vi "02 HEWH First-Hour Rating Test SM1.vi"(0 "Equipment":T6={"COM Port"="COM3", "MW100"="MW100", "AG34970"="A-34972A", "Chamber"="WT500"}, 2 "Semiphore":T1, 5 "Degree Setting":dbl=58.0, 7 "Flow rate setting":dbl=3.0, 11 "Error In":errorcluster) -> (15 "Error Out":errorcluster)   [LabVIEW 2012]
uses:
  EquipReferences.ctl
  HEWH Tank Indicator.ctl
  PowerElements.ctl
  <vilib>/Platform/fileVersionInfo.llb/FileVersionInformation.ctl
  GEA2/HEWH_Mode.ctl
  ChannelSettings.ctl
  ValveBankPositions.ctl
  HEWH Error Enumeration.ctl
  Intellifaucet/Intellfaucet Mode.ctl
  Global HEWH.vi
  <vilib>/Utility/file.llb/Write To Spreadsheet File (string).vi
  <vilib>/Analysis/baseanly.llb/Mean (DBL).vi
  <vilib>/Analysis/NI_AALBase.lvlib
panel:
  in  "Tab Control 4":enum32{"Debug Info", "Version Info"}(tab)
  in  "Stop Logging":bool
  in  "Stop":bool
  in  "StopSerial":bool
  out "Serial Data In":string
  out "Computer Name":string
  out "exe?":bool
  out "Local?":bool
  in  "End Time(s)":dbl=3600.0
  in  "TFall":dbl=25.0
  out "Current Draw Start Time":dbl format="%.2f"
  in  "RTD 2 Downspout offset":dbl
  out "COM Port":refnum<visa-resource-name>
  out "Chanel List":string
  out "Label Array":string[](array[string])
  out "FileVersionInfo Out":T2
  out "Calibration Path 2":path
  out "Calibration File Array":dbl[][](array[numeric])
  out "Com Errs":dbl
  out "Voltage":dbl=240.0
  in  "Stop Test":bool
  out "Ver.":string
  out "DrawCount":i32
  out "POWER":T3
  out "t*=0":dbl format="%.2f"
  out "Elapsed Time (sec)":dbl format="%.2f"
  out "STATUS":string
  in  "Help":bool
  out "Current Log Data":string[][](array[string])
  out "Number of Records":i32
  out "Tank Display":T4 {"TC6" format="%.2g"; "TIN" format="%.2g"; "TOUT" format="%.2g"; "Mean" format="%.2f"; "Std Dev" format="%.2f"; "TC5" format="%.2g"; "TC4" format="%.2g"; "TC3" format="%.2g"; "TC2" format="%.2g"; "TC1" format="%.2g"}
  out "First Time":bool=TRUE
  out "Current State":string
  out "MW100":refnum<visa-resource-name>
  in  "Tab Control 2":enum32{"TEST STATUS", "DATA VIEW"}(tab)
  in  "Tab Control":T5(tab)=enum."External Program Controls"
  in  "Read Config File":bool
  in  "Config Filename":string="HEWH First Hour Rating.ini"
  out "Data Array":string[][](array[string])
  in  "Purge Condition TC":enum16{"TC1", "TC2", "TC3", "TC4", "TC5", "TC6"}(ring)
  out "Serial Port Available?":bool
  in  "Cold Water Available?":bool=TRUE
  in  "T3":u32=500
  in  "T2":u32=150
  in  "Work File Directory":path=path "c:/work"
  out "LAN IP Address":string="192.168.25.3"
  out "Init Complete":bool=TRUE
  in  "T1":u32=1000
  in  "T4":u32=60000
  in  "T5":u32=50
  in  "Purge Guard Time(s)":dbl=300.0
  in  "Data Sample Period(10s)":dbl=10.0
  in  "Purge0 Condition TC":enum16{"TC1", "TC2", "TC3", "TC4", "TC5", "TC6"}(ring)
  in  "PurgreTempLimit":dbl=124.0
  in  "Save File Directory":path=path "c:/data"
  out "FileName":path
  out "Use Agilent?":bool
  out "GEA2 HyperData":bool
  in  "Expansion Tank?":bool=TRUE
  out "Mode":T7=enum."HighDemand"
  out "Set Point":u8=140
  in  "Purgre0TempLim":dbl=124.0
  in  "RTD In Band":dbl=5.0
  in  "Calibration Path":path=path "C:/work/CalibrationFile.csv"
  out "Calibration File?":bool
  out "Monitoring Temps Chart":T8(graph)
  out "Tcs 1-6":dbl[](array[numeric])
  in  "Skip Waiting for Temp":bool
  out "SetPoint":dbl
  out "T2(TankSensor)":dbl
  in  "T2_Threshold":dbl=0.5
  out "Purge Guard Time":dbl=120.0
  out "PurgreTempLimit":dbl=127.0
  out "DrawCount":i32
  out "Purgre0TempLim":dbl=127.0
  out "Purge Condition TC":enum16{"TC1", "TC2", "TC3", "TC4", "TC5", "TC6"}(ring)
  out "Downspount Flow":dbl(graph)
  out "Downspout Flow":dbl=3.8899999999999997
  out "Downspout Temp":dbl=76.8
  out "Temp Band(+/- F)":dbl=50.0
  out "Flow rate Adj":dbl=85.11482133995038
  out "Purge Temperature":dbl(graph)
  out "Temp Adj":dbl
  in  "Skip Purge":bool
  in  "Skip Waiting for Cutout":bool
  in  "meant tank lower lim":dbl=130.0
  in  "mean tank upper lim":dbl=140.0
  out "Ave Tank Temp":dbl format="%0.2f"
  out "Tc_1":dbl
  in  "Tc1 UL":dbl=140.0
  in  "Tc1 LL":dbl=130.0
  in  "Skip Waiting for Temp 3":bool
  out "Tcs 1-6, Ave. 3":dbl[](array[numeric])
  out "Temps Chart 2":T9(graph)
  out "T_Ave":dbl
  in  "Temp Decline Hystersis":dbl=0.2
  out "T_Ave_Max":dbl
  out "LastDraw":bool=TRUE
  in  "Begin Draw":bool
  out "RTD OUT":dbl(graph)
  out "Last T*min":dbl
  out "Special Last Draw":bool
  out "Discard Last Draw":bool
  out "T*Ave":dbl
  out "T*min":dbl
  out "M*(Gallons)":dbl
  out "T*max":dbl
  out "FlowMeter During Draw":dbl(graph)
  out "Flow":dbl=3.8899999999999997
  out "RTD_IN Value":dbl
  out "Tin Fault":bool
  out "Temp Adj Draw":dbl
  out "Flow Adj Draw":dbl
  out "Iteration":i32
  out "Drawing":bool=TRUE
  out "ETime":dbl format="%.2f"
  in  "K(0.1)":dbl=0.2
  in  "Flow Adjust Time (3s)":dbl=1.5
  out "WattHours":dbl
  out "Error History":string[](array[string])
  out "Com History":string[](array[string])
  out "Test Data":dbl[][](array[numeric])
  out "Executaion Sequence":string[](array[string])
  out "Error Datalogging":errorcluster={"status"=TRUE, "code"=-1073807346, "source"="VISA Read in Gather Test Data.vi"}
  out "Error Serial":errorcluster
  in  "Tab Control 3":enum32{"Temperature", "Power", "Gallons"}(tab)
  out "Temps":T8(graph) caption="Waveform Chart"
  out "Watt Chart":T10(graph)
  out "Gallons Chart":dbl(graph)
  # "FIRST-HOUR RATING TEST"
  # "Offset added to initial draw for initial value\nin Draw."
  # "wait for purge condition:\npower is off or...\nend of time is near or...\npurge condition tc > purge temp limit \nnote temp limit different between first and subsequent runs."
  # "Wait for Cutout..."
  # "Input relays don't detect that UE or LE are on, and Power reading <\nCompressor LL (0.35 kW currently)"
  # "This draw initiation criterion for heat pump\nwater heaters that use supplemental resistive\nheating, however, shall only apply when\nthe water located above the thermostat at\ncut-out is heated to 135 °F±5 °F (57.2 °C±2.8\n°C)."
  # "WAIT FOR TOP HEATER AND COMP OFF."
  # "T*max is max ave temp"
  # "(For Last Draw, If after 30 sec, T< last tmin, stop and discard measurements, else continue)"
  # "Record output water temp after 15 secs, and at 5 sec intervals thereafter\nMonitor inlet water temp, must be 58 +/- 2 F\nTerminate draw when output temp = T*max -25F, record T*min"
  # "Terminate draw.  Record Tmin*, Tmax*, Tave* and M*"
  # "(For Last Draw, If after 30 sec, T< last tmin, stop and discard measurements, else continue)"
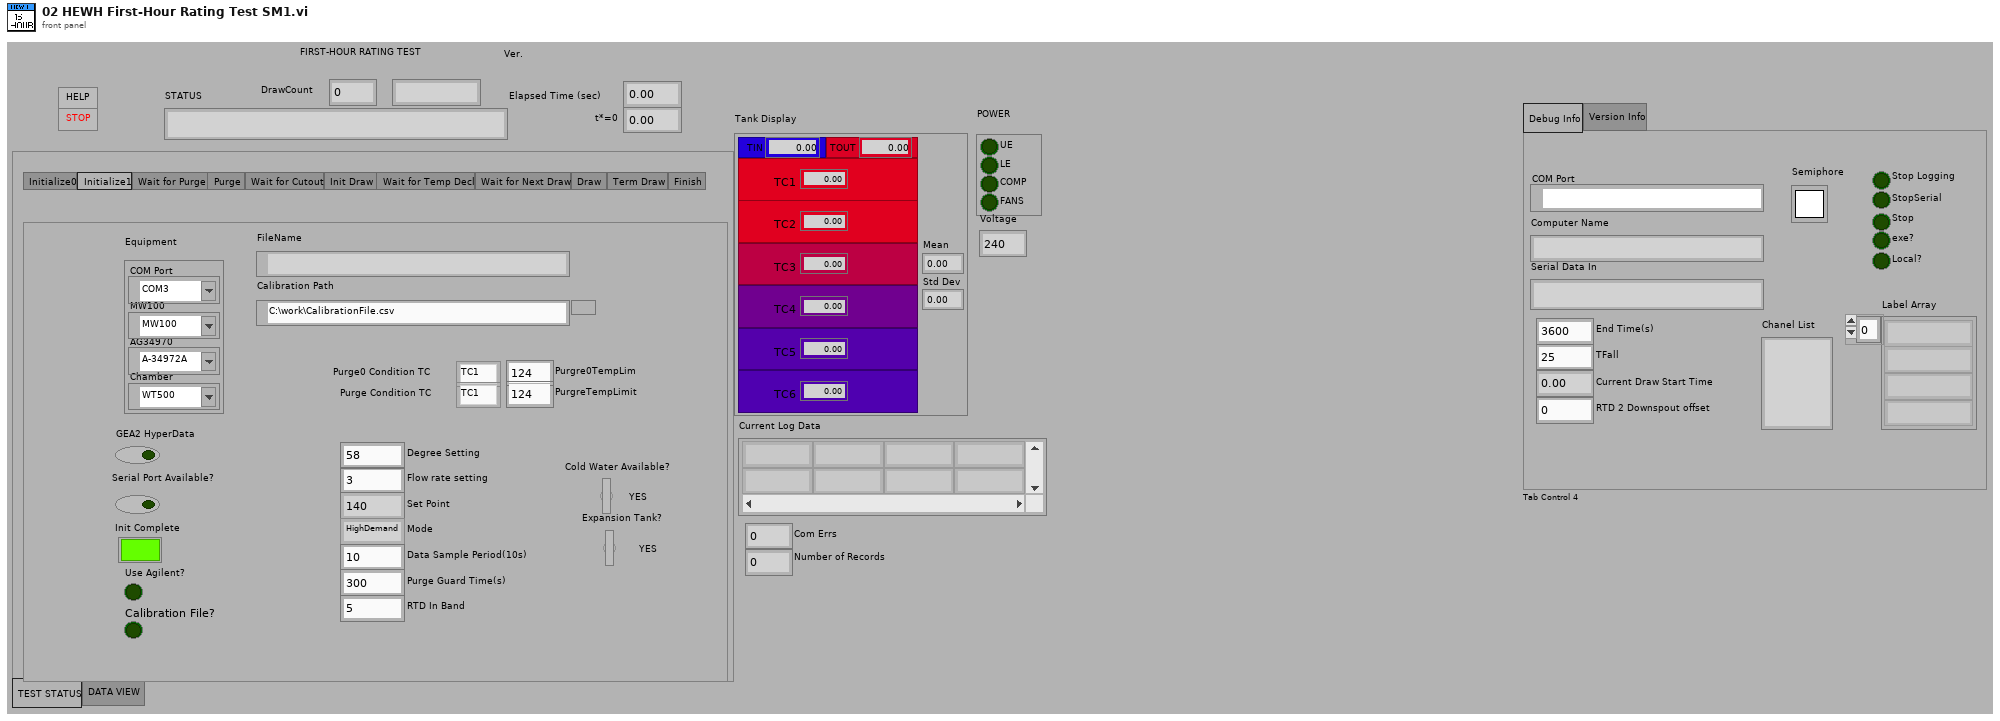
[diagram p1: front panel]
types:
  T1 = typedef "Semaphore RefNum" = refnum<k1>
  T2 = typedef "FileVersionInformation.ctl" = cluster{"FileVersion":string, "ProductName":string, "InternalName":string, "CompanyName":string, "LegalCopyright":string, "FileDescription":string}
  T3 = typedef "PowerElements.ctl" = cluster{"UE":bool, "LE":bool, "COMP":bool, "FANS":bool}
  T4 = typedef "HEWH Tank Indicator.ctl" = cluster{"TC1-D":bool, "TC2-D":bool, "TC3-D":bool, "TC4-D":bool, "TC5-D":bool, "RTD_IN":bool, "RTDOUT":bool, "TC1":dbl, "TC2":dbl, "TC3":dbl, "TC4":dbl, "TC5":dbl, "TIN":dbl, "TOUT":dbl, "Std Dev":dbl, "Mean":dbl, "TC6-D":bool, "TC6":dbl}
  T5 = enum32{"Initialize0", "External Program Controls", "External Program Controls 2", "Program Controls", "Feedback", "Init Draw", "Feedback 3", "Feedback 4", "Draw", "Feedback 5", "Feedback 6"}
  T6 = typedef "EquipReferences.ctl" = cluster{"COM Port":refnum<visa-resource-name>, "MW100":refnum<visa-resource-name>, "AG34970":refnum<visa-resource-name>, "Chamber":refnum<visa-resource-name>}
  T7 = typedef "HEWH_Mode.ctl" = enum16{"Hybrid", "StdElectric", "eHeat", "HighDemand", "Vacation"}
  T8 = cluster{"Tc Tree[0]":dbl, "Tc Tree[1]":dbl, "Tc Tree[2]":dbl, "Tc Tree[3]":dbl, "Tc Tree[4]":dbl, "Tc Tree[5]":dbl}[]
  T9 = cluster{"[0]":dbl, "[1]":dbl, "[2]":dbl, "[3]":dbl, "[4]":dbl, "[5]":dbl, "[6]":dbl}[]
  T10 = cluster{"[0]":dbl, "[1]":dbl, "[2]":dbl, "[3]":dbl, "[4]":dbl, "[5]":dbl}[]
  T11 = enum32{"invalid app kind", "Development System", "Run Time System", "Student Edition", "Embedded LabVIEW", "Evaluation", "Custom"}
  T12 = typedef "ValveBankPositions.ctl" = enum16{"Heating", "Purge", "Resting", "Draw"}
  T13 = typedef "HEWH Error Enumeration.ctl" = enum16{"No Error", "GEA2 Send ACK Mismatch", "GEA2 STX", "GEA2 ETX", "GEA2 CRC Mismatch", "GEA2 ReadACK", "RTD In Range Error", "Fail Mean Tank Temp", "No Flow Config Data Found", "Failed Flow During Purge", "Temp During Purge", "Confirm IF Stop Fail", "Init Draw: TC_1 Out of Range", "Flow = 0 During Draw after 20s"}
  T14 = typedef "Intellfaucet Mode.ctl" = enum16{"Adjust Temp", "Adjust Flow", "Start Flow", "Stop Flow"}
  T15 = typedef "TestedFlowratesScenarios.ctl" = enum16{"DRK500,Station1", "DRK375,Lab", "SRK500,Station1,5GPM FR", "DRK375,STATION3,1/2\"HOSE", "DRK500,Station1,downspout", "DRK375,Station3,thruEcocute", "DRK375,Station3,purge", "Build2,2B,Purge", "Global, Purge", "Global, Tank"}
  T16 = cluster{"Serial Port Available?":bool, "Cold Water Available?":bool, "TempErLimit":dbl, "Temp Decline Hystersis":dbl, "Target IP Address":string, "Draw Tesw Condition":T15}
  T17 = cluster{"Degree Setting":dbl, "Flow rate setting":dbl, "TFall":dbl, "End Time(s)":dbl, "Tc1 LL":dbl, "Tc1 UL":dbl}
  T18 = cluster{"No Serial  Sample Period(s)":dbl, "T5":u32, "T4":u32, "T1":u32, "T2":u32, "T3":u32}
  T19 = typedef "Cluster Purge Settings.ctl" = cluster{"Temp SettleTimeLimit(S)":dbl, "Steady State Persist Time(mS)":u32, "Purge Min Time":i32, "Flow SettleTimeLimit(S)":dbl, "Flow Adjust Time (3s)":dbl, "Flow Band (+/-GPM)":dbl, "Proportional Control Adjust Rate":dbl}
  T20 = cluster{"PurgreTempLimit":dbl, "Purge Condition TC":enum16{"TC1", "TC2", "TC3", "TC4", "TC5", "TC6"}, "Purgre0TempLim":dbl, "Purge Guard Time(s)":dbl}
  T21 = enum16{"Computation Start", "Computation stop", "Reset Computation", "Clear Computation"}[]
  T22 = cluster{"Tc Tree[0]":dbl, "Tc Tree[1]":dbl, "Tc Tree[2]":dbl, "Tc Tree[3]":dbl, "Tc Tree[4]":dbl, "Tc Tree[5]":dbl}
  T23 = cluster{"[0]":dbl, "[1]":dbl, "[2]":dbl, "[3]":dbl, "[4]":dbl, "[5]":dbl, "[6]":dbl}
  T24 = typedef "PowerData.ctl" = cluster{"Voltage":dbl, "Current":dbl, "Power":dbl, "WattHours":dbl}
  T25 = cluster{"[0]":dbl, "[1]":dbl, "[2]":dbl, "[3]":dbl, "[4]":dbl, "[5]":dbl}
  T26 = typedef "ChannelSettings.ctl" = u32
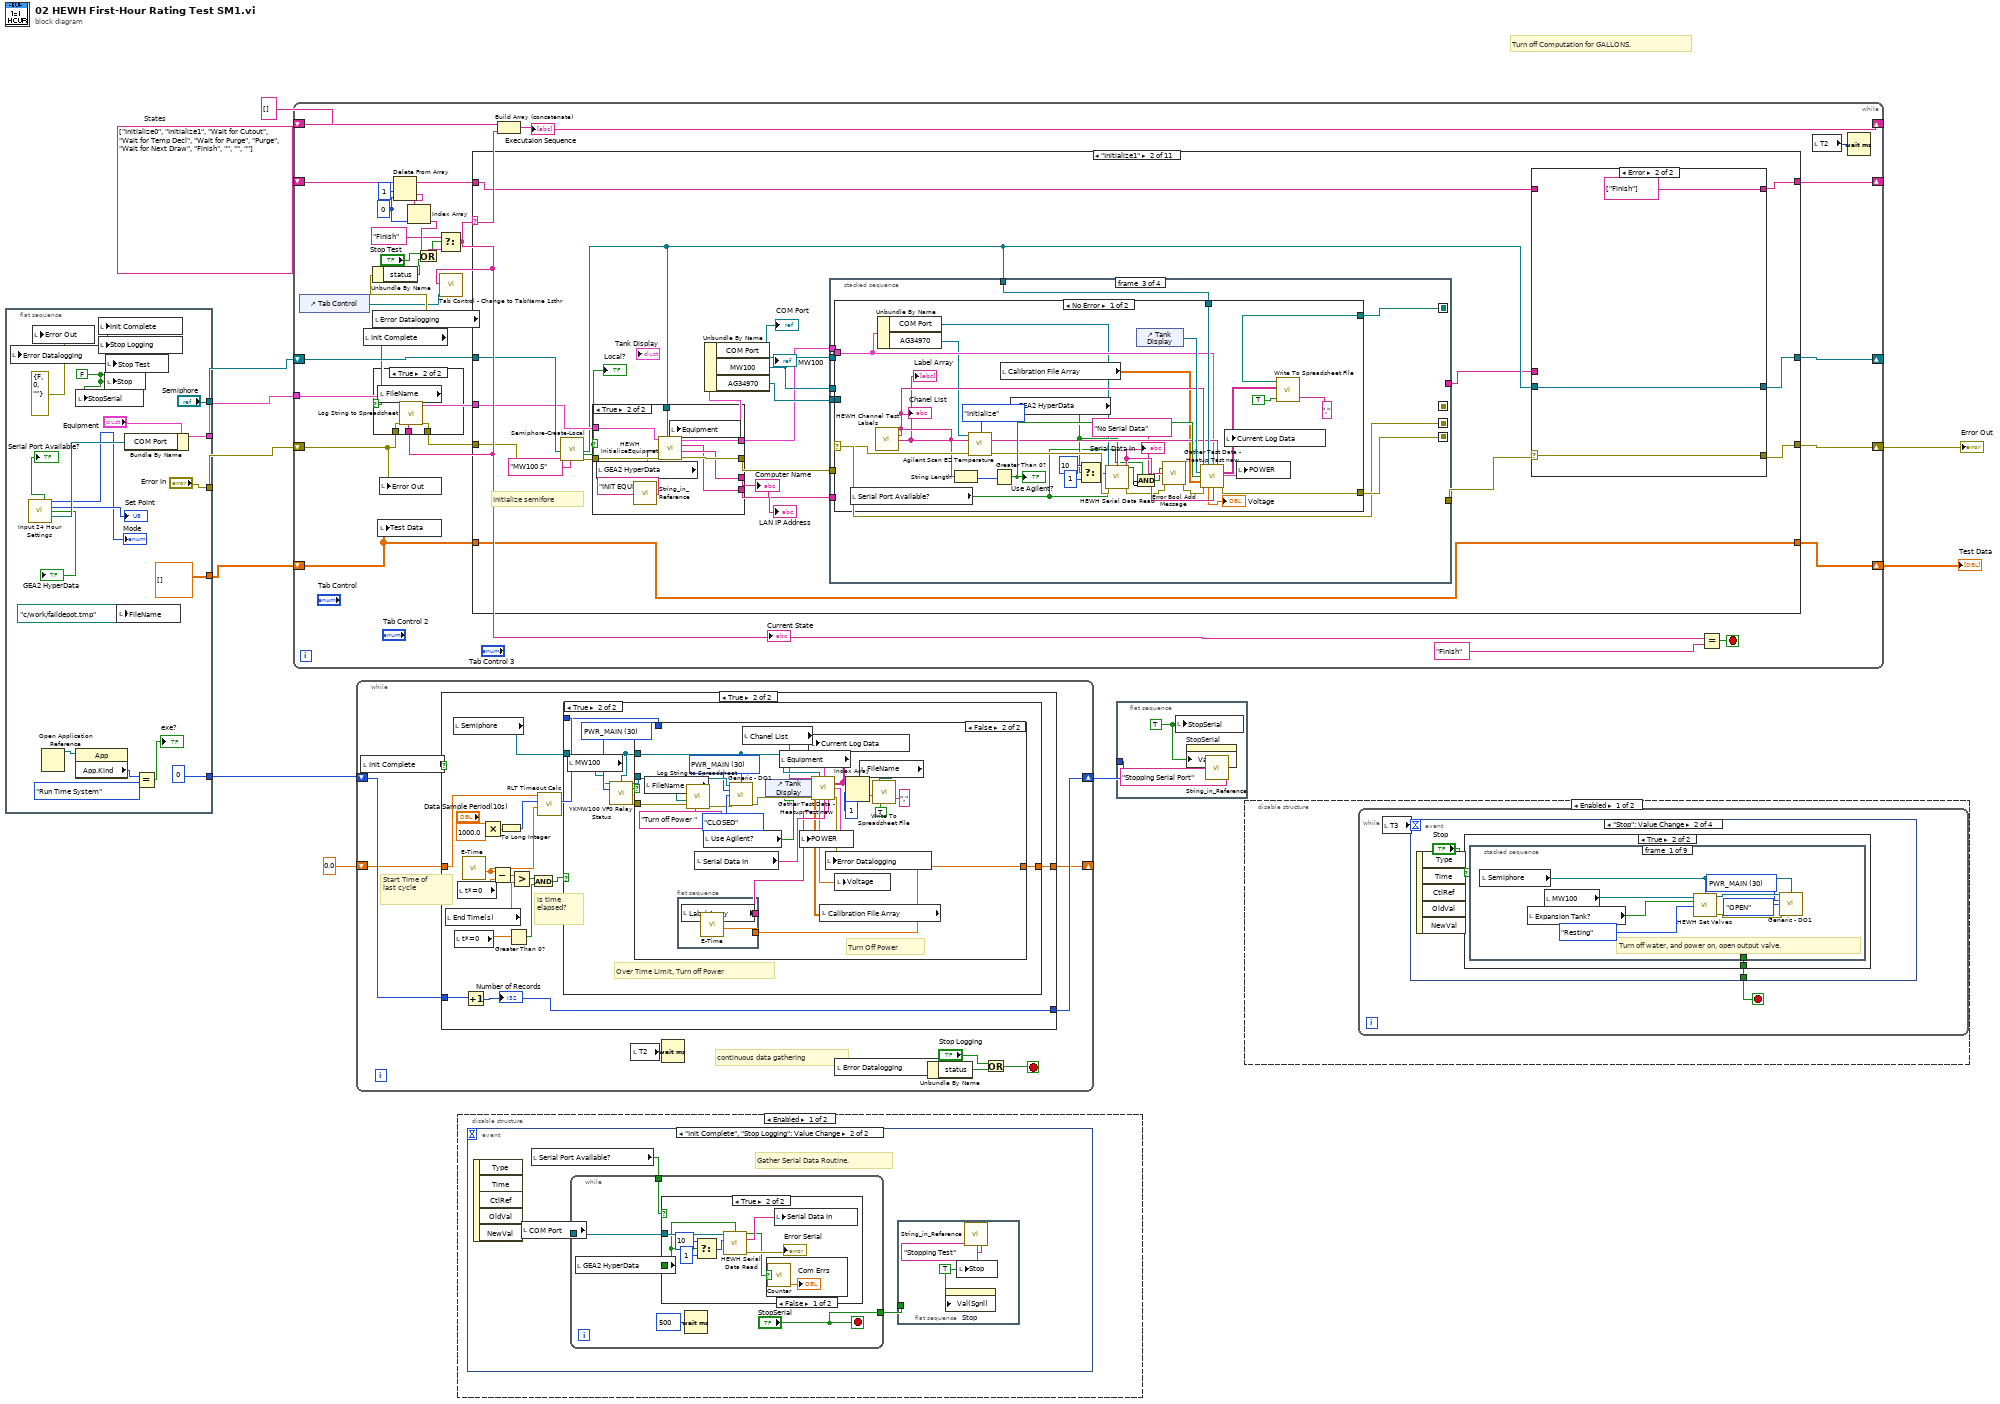
[diagram p0: block diagram]
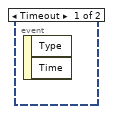
[diagram p2: hidden frame]
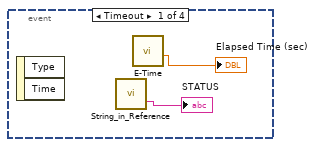
[diagram p6: hidden frame]
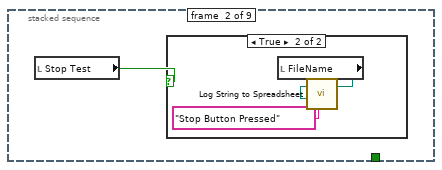
[diagram p8: hidden frame]
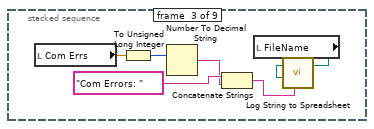
[diagram p10: hidden frame]
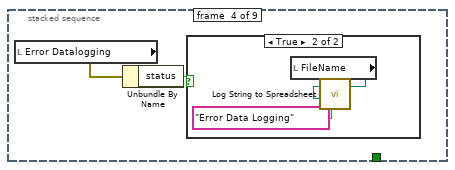
[diagram p11: hidden frame]
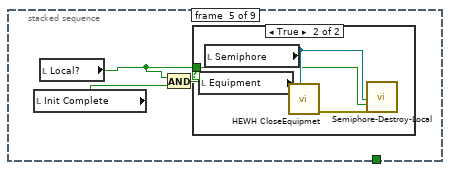
[diagram p13: hidden frame]
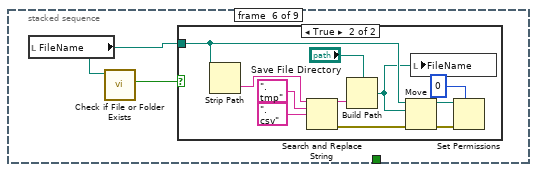
[diagram p15: hidden frame]
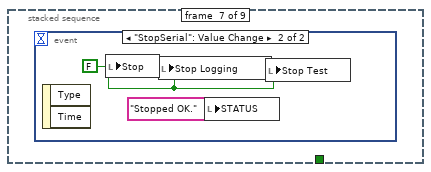
[diagram p17: hidden frame]
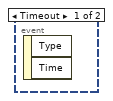
[diagram p18: hidden frame]
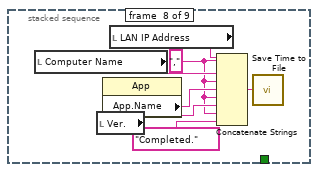
[diagram p19: hidden frame]
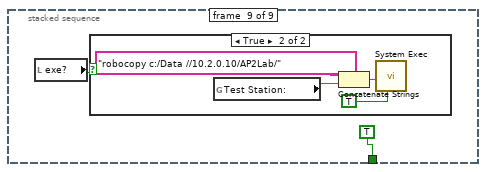
[diagram p20: hidden frame]
diagram:
  w1 = string[] ["Initialize0", "Initialize1", "Wait for Cutout", "Wait for Temp Decl", "Wait for Purge", "Purge", "Wait for Next Draw", "Finish", "", "", ""]  # States
  # "Turn off Computation for GALLONS."
  n1 = flat-sequence {
    tunnel: ["Semiphore"] -> w5
    tunnel: [w25] -> w6
    tunnel: ["Error In"] -> w4
    tunnel: [dbl[][] []] -> w3
    tunnel: [0 ("milliseconds to wait")] -> w2
    frame #0 {
      w17 = errorcluster {"status"=FALSE, "code"=0, "source"=""} ("Error Datalogging")
      w28 = FALSE ("First Time 2")
      n2 = local write "Error Datalogging"(w17) -> ()
      n3 = call "Input 24 Hour Settings.vi"() -> ("Serial Port Available?"=→"Serial Port Available?":bool, "GEA2 Set Mode Out"=→"Mode":T7, "Set PointOut"=→"Set Point":u8, "GEA2 HyperData Out"=→"GEA2 HyperData":bool, "COM Port Out"=w26:refnum<visa-resource-name>)  [unwired: 10 in, 1 out]
      n4 = local write "Error Out"(w17) -> ()
      n5 = Open Application Reference() -> (3:w16:refnum<vi>)  [unwired: 4 in, 1 out]
      n6 = local write "StopSerial"(w28) -> ()
      n7 = property class="App"(reference=w16) -> ("App.Kind"=w15:T11)  [unwired: 1 in, 2 out]
      n8 = local write "Init Complete"(w28) -> ()
      n9 = local write "Stop Logging"(w28) -> ()
      n10 = local write "Stop"(w28) -> ()
      n11 = local write "Stop Test"(w28) -> ()
      n12 = local write "FileName"(path "c:/work/faildepot.tmp" ("FileName")) -> ()
      n13 = Bundle By Name(cluster="Equipment", "COM Port"=w26) -> (w25:T6)
      n14 = Equal?(x=w15, y=T11."Run Time System" ("Application:Kind")) -> (x = y?=→"exe?":bool)
    }
  }
  n15 = while {
    shift-right: [w54] -> _
    shift-left: w1 -> [w57]
    shift-right: [w52] -> w9
    shift-left: w4 -> [w39]
    tunnel: w6 -> [w48]
    shift-right: [w47] -> w11
    shift-left: w3 -> [w46]
    shift-right: [w45] -> _
    shift-left: w5 -> [w49]
    shift-right: [w41] -> _
    shift-left: string[] [] -> [w42]
    stop <- w51 stop-if-true
    w44 = 0 ("index")
    n16 = control-ref of="Tab Control"() -> (w30:refnum<vi>)
    n17 = local read "Init Complete"() -> (w40:bool)
    n18 = local read "Error Datalogging"() -> (w33:errorcluster)
    n19 = Unbundle By Name(w33) -> ("status"=w32:bool)
    n20 = local write "Test Data"(w46) -> ()
    n21 = local write "Error Out"(w39) -> ()
    n22 = Delete From Array(array=w57, length=1, index=w44) -> (deleted portion=w55:string[], array with subset deleted=w53:string[])
    n23 = Index Array(array=w55, index=w44) -> (element=w36:string)
    n24 = Or(x="Stop Test", y=w32) -> (x .or. y?=w31:bool)
    n25 = Select(t="Finish", s=w31, f=w36) -> (s? t:f=w37:string)
    "Current State" <- w37
    n26 = case shown="True" w40 {
      tunnel: w39 -> [w58 w61]
      tunnel: [w58 w60] -> w38
      tunnel: w37 -> [_ w59]
      frame False {
      }
      frame True {
        n27 = local read "FileName"() -> (w62:path)
        n28 = call "Log String to Spreadsheet.vi"("String"=w59, "error in (no error)"=w61, "FileName"=w62) -> ("error out"=w60:errorcluster)  [unwired: 8 in]
      }
    }
    n29 = call "Tab Control - Change to TabName 1sthr.vi"("Label.Text"=w37, "TabCtl Refnum"=w30) -> ()  [unwired: 9 in]
    n30 = case shown="\"Initialize1\"" w37 {
      tunnel: [w77 w164 w327 w485 w522 w617 w686 w807 w883 w1015 w1058] -> w54
      tunnel: w53 -> [w76 w165 w328 w483 w520 w615 w687 _ w880 w1016 w1057]
      tunnel: [w75 w163 w326 w484 w521 w616 w684 w811 w881 w1014 w1047] -> w52
      tunnel: w38 -> [w72 w158 w317 w479 w515 w602 w683 w809 w886 w1007 w1047]
      tunnel: w49 -> [w74 w162 w330 w471 w518 w612 w681 w806 w889 w1003 w1046]
      tunnel: w48 -> [_ w161 w329 w472 _ w611 _ _ w884 _ w1056]
      tunnel: [w73 w160 w331 w482 w519 w614 w688 w810 w887 w1013 w1055] -> w47
      tunnel: w46 -> [w73 w160 w331 w482 w519 w614 w688 w810 w887 w1012 w1055]
      tunnel: [w74 w159 w330 w471 w518 w612 w681 w806 w885 w1003 w1046] -> w45
      frame "Initialize0" {
        # "Flow Loop Time"
        # "1 Min Between Samps in spec."
        # "UI Refresh Rate"
        # "Loop Delays, prevent overwork Machine"
        # "Sample Period for Decision Data"
        n31 = Current VI's Path() -> (path=w78:path)
        n32 = call "This VIs Path.vi"("path"=w78, "error in (no error)"=w72) -> ("current path"=w83:path, "File Version Info"=→"Ver.":string, "FileVersionInfo Out"=→"FileVersionInfo Out":T2, "error out"=w79:errorcluster)  [unwired: 9 in, 1 out]
        n33 = Build Path(base path=w83, name or relative path="Config Filename") -> (appended path=w80:path)
        n34 = case shown="False" "Read Config File" {
          tunnel: w80 -> [_ w114]
          tunnel: ["Flow rate setting" w110] -> w71
          tunnel: w79 -> [w103 w109]
          tunnel: [w103 w108] -> w68
          tunnel: ["Degree Setting" w105] -> w69
          frame False {
          }
          frame True {
            n35 = call "Config File First Hour.vi"("Config File Path"=w114, "Error In"=w109) -> ("Test Condition Settings Cluster"=w113:T16, "DOE Test Spec Settings Cluster"=w112:T17, "Timing Cluster"=w111:T18, "Purge Settings Cluster"=w106:T19, "Purge Condition Settings Cluster"=w107:T20, "Error Out"=w108:errorcluster)  [unwired: 8 in]
            n36 = stacked-sequence {
              tunnel: w113 -> [w119 _ _ _ _ _]
              tunnel: w112 -> [_ w126 _ _ _ _]
              tunnel: w111 -> [_ _ w133 _ _ _]
              tunnel: [_ w121 _ _ _ _] -> w110
              tunnel: w108 -> [_ _ _ _ _ w140]
              tunnel: w107 -> [_ _ _ _ w135 _]
              tunnel: w106 -> [_ _ _ w134 _ _]
              tunnel: [_ w120 _ _ _ _] -> w105
              frame #0 {
                n37 = Unbundle(w119) -> ("Serial Port Available?"=w118:bool, "Cold Water Available?"=w117:bool, "Temp Decline Hystersis"=w116:dbl, "Target IP Address"=w115:string)  [unwired: 2 out]
                n38 = local write "Cold Water Available?"(w117) -> ()
                n39 = local write "Serial Port Available?"(w118) -> ()
                n40 = local write "Temp Decline Hystersis"(w116) -> ()
                n41 = local write "LAN IP Address"(w115) -> ()
              }
              frame #1 {
                n42 = Unbundle(w126) -> ("Degree Setting"=w120:dbl, "Flow rate setting"=w121:dbl, "TFall"=w125:dbl, "End Time(s)"=w124:dbl, "Tc1 LL"=w123:dbl, "Tc1 UL"=w122:dbl)
                n43 = local write "Flow rate setting"(w121) -> ()
                n44 = local write "Degree Setting"(w120) -> ()
                n45 = local write "End Time(s)"(w124) -> ()
                n46 = local write "Tc1 UL"(w122) -> ()
                n47 = local write "Tc1 LL"(w123) -> ()
                n48 = local write "TFall"(w125) -> ()
              }
              frame #2 {
                n49 = Unbundle(w133) -> ("No Serial  Sample Period(s)"=w132:dbl, "T5"=w127:u32, "T4"=w128:u32, "T1"=w129:u32, "T2"=w130:u32, "T3"=w131:u32)
                n50 = local write "Data Sample Period(10s)"(w132) -> ()
                n51 = local write "T1"(w129) -> ()
                n52 = local write "T2"(w130) -> ()
                n53 = local write "T3"(w131) -> ()
                n54 = local write "T5"(w127) -> ()
                n55 = local write "T4"(w128) -> ()
              }
              frame #3 {
                n56 = Unbundle By Name(w134) -> ()  [unwired: 2 out]
              }
              frame #4 {
                n57 = Unbundle(w135) -> ("PurgreTempLimit"=w136:dbl, "Purge Condition TC"=w137:enum16{"TC1", "TC2", "TC3", "TC4", "TC5", "TC6"}, "Purgre0TempLim"=w138:dbl, "Purge Guard Time(s)"=w139:dbl)
                n58 = local write "Purge0 Condition TC"(w137) -> ()
                n59 = local write "Purge Guard Time(s)"(w139) -> ()
                n60 = local write "PurgreTempLimit"(w136) -> ()
                n61 = local write "Purgre0TempLim"(w138) -> ()
              }
              frame #5 {
                n62 = case shown="Error" w140 {
                  frame No Error {
                  }
                  frame Error {
                    n63 = call <vilib>:"Simple Error Handler.vi"("error in (no error)"=errorcluster {"status"=TRUE, "code"=-600, "source"="Config File Error"}) -> ()  [unwired: 4 in, 5 out]
                    n64 = Stop(stop? (T)=TRUE) -> ()
                  }
                }
              }
            }
          }
        }
        n65 = stacked-sequence {
          tunnel: w71 -> [_ _ _ _ _ _ _]
          tunnel: w69 -> [_ w87 _ _ _ _ _]
          frame #0 {
            # "Clear Charts."
            n66 = property on="Monitoring Temps Chart" class="WFChart (strict)"("History Data"=T8 []) -> ()  [unwired: 2 in, 2 out]
            "DrawCount" <- 0
          }
          frame #1 {
            n67 = local write "Temp Adj Draw"(w87) -> ()
            "t*=0" <- 0.0 ("t*=0")
          }
          frame #2 {
            w89 = dbl[] [] ("History Data")
            n68 = property on="Downspount Flow" class="WFChart (strict)"("History Data"=w89) -> ()  [unwired: 2 in, 2 out]
            n69 = property on="RTD OUT" class="WFChart (strict)"("History Data"=w89) -> ()  [unwired: 2 in, 2 out]
            n70 = property on="FlowMeter During Draw" class="WFChart (strict)"("History Data"=w89) -> ()  [unwired: 2 in, 2 out]
            n71 = property on="Purge Temperature" class="WFChart (strict)"("History Data"=w89) -> ()  [unwired: 2 in, 2 out]
            n72 = property on="Gallons Chart" class="WFChart (strict)"("History Data"=w89) -> ()  [unwired: 2 in, 2 out]
            n73 = property on="FlowMeter During Draw" class="WFChart (strict)"("History Data"=w89) -> ()  [unwired: 2 in, 2 out]
          }
          frame #3 {
            w92 = T8 [] ("History Data")
            n74 = property on="Watt Chart" class="WFChart (strict)"("History Data"=T10 []) -> ()  [unwired: 2 in, 2 out]
            n75 = property on="Temps Chart 2" class="WFChart (strict)"("History Data"=T9 []) -> ()  [unwired: 2 in, 2 out]
            n76 = property on="Temps" class="WFChart (strict)"("History Data"=w92) -> ()  [unwired: 2 in, 2 out]
            n77 = property on="Monitoring Temps Chart" class="WFChart (strict)"("History Data"=w92) -> ()  [unwired: 2 in, 2 out]
          }
          frame #4 {
            w93 = FALSE ("BottomHeater")
            n78 = local write "Skip Waiting for Temp"(w93) -> ()
            n79 = local write "Skip Waiting for Cutout"(w93) -> ()
            n80 = local write "LastDraw"(w93) -> ()
            n81 = local write "Help"(w93) -> ()
            n82 = local write "Serial Data In"("0:0:0 UE 24 LE 24 COMP 0 FAN1 0 FAN2 0 SP:0 0 0 0 0 0 C030" ("trimmed string")) -> ()
            n83 = local write "Drawing"(w93) -> ()
            n84 = local write "Tin Fault"(w93) -> ()
            n85 = local write "POWER"(T3 {"UE"=FALSE, "LE"=FALSE, "COMP"=FALSE, "FANS"=FALSE} ("POWER 2")) -> ()
            n86 = local write "Begin Draw"(w93) -> ()
            "First Time" <- TRUE ("First Time")
            "Special Last Draw" <- w93
            "Discard Last Draw" <- w93
          }
          frame #5 {
            n87 = local write "RTD_IN Value"(0.0 ("RTD_IN Value")) -> ()
            n88 = Select(t="RTD In Band", s="Cold Water Available?", f=55.0) -> (s? t:f=→"Temp Band(+/- F)":dbl)
          }
          frame #6 {
            n89 = call "HEWH Config Read.vi"() -> ()  [unwired: 14 in, 2 out]
          }
        }
        n90 = call "Calibration File Check.vi"("error in (no error)"=w68, "Calibration Path"="Calibration Path") -> ("error out"=w67:errorcluster, "Calibration Path"=→"Calibration Path 2":path, "Calibration File Array"=→"Calibration File Array":dbl[][], "Complete File?"=→"Calibration File?":bool)  [unwired: 6 in]
        n91 = case shown="No Error" w67 {
          selector: w67 -> [w144 w146]
          tunnel: [w143 string[] ["Finish"] ("States")] -> w77
          tunnel: [w144 w146] -> w75
          tunnel: w76 -> [w143 _]
          frame No Error {
          }
          frame Error {
          }
        }
      }
      frame "Initialize1" {
        # "Initialize semifore"
        n92 = call "Semiphore-Create-Local.vi"("Semiphore"=w162, "error in (no error)"=w158, "name (unnamed)"="MW100 S") -> ("semaphore"=w152:T1, "Local?"=w166:bool, "error out"=w167:errorcluster)  [unwired: 14 in]
        "Local?" <- w166
        n93 = case shown="True" w166 {
          tunnel: w167 -> [w306 w309]
          tunnel: [w305 w314] -> w153
          tunnel: [w306 w315] -> w156
          tunnel: w161 -> [w305 w308]
          tunnel: w152 -> [_ w310]
          tunnel: [w304 w312] -> w150
          tunnel: [w303 w311] -> w157
          frame False {
            n94 = call "IP and Computer Name.vi"() -> ("IP Address"=w303:string, "Computer Name"=w304:string)  [unwired: 10 in]
          }
          frame True {
            n95 = local read "GEA2 HyperData"() -> (w307:bool)
            n96 = call "String_in_Reference.vi"("String"="INIT EQUIP") -> ()  [unwired: 18 in, 1 out]
            n97 = call "HEWH InitializeEquipmet.vi"("Semiphore"=w310, "Error In"=w309, "GEA2?"=w307, "Equipment"=w308) -> ("Error Out"=w315:errorcluster, "Computer Name"=w312:string, "LAN IP Address"=w311:string, "Equipment Out"=w314:T6)  [unwired: 4 in]
            n98 = local write "Equipment"(w314) -> ()
          }
        }
        "LAN IP Address" <- w157
        "Computer Name" <- w150
        n99 = Unbundle By Name(w153) -> ("COM Port"=w147:refnum<visa-resource-name>, "MW100"=w155:refnum<visa-resource-name>, "AG34970"=w154:refnum<visa-resource-name>)
        "MW100" <- w155
        "COM Port" <- w147
        n100 = stacked-sequence {
          seq-local: [_ w198 _ _] -> [_ _ w235 _]
          seq-local: [w169 _ _ _] -> [_ w189 _ _]
          seq-local: [_ _ w237 _] -> [_ _ _ w274]
          seq-local: [_ w201 _ _] -> [_ _ w236 _]
          tunnel: [_ _ _ w276] -> w151
          tunnel: w150 -> [_ w200 _ _]
          tunnel: w156 -> [w171 _ _ _]
          tunnel: w155 -> [w179 _ _ w273]
          tunnel: w154 -> [_ _ w240 _]
          tunnel: w153 -> [_ _ w239 _]
          tunnel: w152 -> [w170 _ w238 w275]
          tunnel: [_ w202 _ _] -> w149
          tunnel: w147 -> [w172 w188 _ _]
          frame #0 {
            # "Set Valves."
            n101 = local write "Semiphore"(w170) -> ()
            n102 = call "HEWH Set Valves.vi"("VISA session"=w179, "Semiphore"=w170, "Expansion Tank?"="Expansion Tank?", "Valve Bank Setting"=ValveBankPositions."Heating", "Error In"=w171) -> ("dup VISA session"=w177:refnum<visa-resource-name>, "Error Out"=w178:errorcluster)  [unwired: 9 in]
            n103 = local read "GEA2 HyperData"() -> (w168:bool)
            n104 = call "HEWH Totalize Flow Control.vi"("VISA session"=w177, "Semiphore"=w170, "Totalize Flow"=FALSE, "error in (no error)"=w178) -> ("error out"=w173:errorcluster)  [unwired: 10 in, 1 out]
            n105 = case shown="True" w168 {
              tunnel: w173 -> [w180 w185]
              tunnel: w172 -> [_ w184]
              tunnel: [w180 w183] -> w169
              frame False {
              }
              frame True {
                n106 = local read "Set Point"() -> (w181:u8)
                n107 = local read "Mode"() -> (w182:T7)
                n108 = call "HEWH GEA2 Set Tank Mode and Temp.vi"("ComPort"=w184, "Mode"=w182, "Set Point"=w181, "Error In"=w185) -> ("Error Out"=w183:errorcluster)  [unwired: 9 in, 2 out]
              }
            }
          }
          frame #1 {
            # "Initialize Data file ."
            n109 = local read "Set Point"() -> (w193:u8)
            n110 = local read "Mode"() -> (w187:T7)
            n111 = property on="Mode" class="Enum (strict)"() -> ("Strings []"=w191:string[])  [unwired: 2 in, 2 out]
            n112 = To Long Integer(number=w187) -> (32bit integer=w192:i32)
            n113 = Index Array(array=w191, index=w192) -> (element=w197:string)
            n114 = Number To Decimal String(number=w193) -> (decimal integer string=w195:string)  [unwired: 1 in]
            n115 = Concatenate Strings("Mode:" ("Test_Type In:"), w197, " Tset:" ("Test_Type In:"), w195) -> (w194:string)
            n116 = case shown="\"Hybrid\", Default" w187 {
              tunnel: ["SE" ("Mode:") "EH" ("Mode:") "HD" ("Mode:") "HY" ("Mode:")] -> w186
              frame "StdElectric" {
              }
              frame "eHeat" {
              }
              frame "HighDemand" {
              }
              frame "Hybrid", Default {
              }
            }
            n117 = case shown="No Error" w189 {
              selector: w189 -> [_ w233]
              tunnel: [w224 string[][] [] ("Data Array")] -> w205
              tunnel: [w213 path "" ("FileName")] -> w201
              tunnel: w200 -> [w223 _]
              tunnel: "tmp" ("File Extension:") -> [w219 _]
              tunnel: w189 -> [w218 _]
              tunnel: [w216 w233] -> w198
              tunnel: w194 -> [w217 _]
              tunnel: w188 -> [w214 _]
              tunnel: w186 -> [w212 _]
              frame No Error {
                n118 = local read "FileVersionInfo Out"() -> (w221:T2)
                n119 = Unbundle By Name(w221) -> ("FileVersion"=w220:string)  [unwired: 1 out]
                n120 = local read "GEA2 HyperData"() -> (w210:bool)
                n121 = call "Data_File_Init.vi"("Data File Directory"="Work File Directory", "Test_Name In:"="FIRST", "Version In:"=w220, "Computer Name In:"=w223, "error in (no error)"=w218, "File Extension:"=w219, "Ambient Temp / RH:"=w217, "Mode:"=w212) -> ("FileName"=w213:path, "Data Array"=w224:string[][], "error out"=w215:errorcluster)  [unwired: 5 in]
                "FileName" <- w213
                "Data Array" <- w224
                n122 = case shown="True" w210 {
                  tunnel: [w225 w231] -> w216
                  tunnel: w215 -> [w225 w229]
                  tunnel: w214 -> [_ w228]
                  tunnel: w213 -> [_ w227]
                  frame False {
                  }
                  frame True {
                    n123 = call "GEA2_RQST_SOFTWARE_VER.vi"("ComPort"=w228, "Error In"=w229) -> ("Software Version"=w226:string, "Error Out"=w230:errorcluster)  [unwired: 10 in, 2 out]
                    n124 = call "Log String to Spreadsheet.vi"("String"=w226, "error in (no error)"=w230, "FileName"=w227) -> ("error out"=w231:errorcluster)  [unwired: 8 in]
                  }
                }
              }
              frame Error {
              }
            }
            n125 = Array To Spreadsheet String(delimiter (Tab)=",", array=w205, 3:"%s" ("format string")) -> (spreadsheet string=w202:string)
          }
          frame #2 {
            n126 = case shown="No Error" w235 {
              selector: w235 -> [w271 w272]
              tunnel: w240 -> [_ _]
              tunnel: w239 -> [w259 _]
              tunnel: w238 -> [w264 _]
              tunnel: [w256 w272] -> w237
              tunnel: w236 -> [w252 _]
              frame No Error {
                n127 = local read "Serial Port Available?"() -> (w242:bool)
                n128 = call "HEWH Channel Test Labels.vi"() -> ("Chanel List"=w265:string, "Label List"=w262:string[])  [unwired: 13 in, 1 out]
                "Chanel List" <- w265
                "Label Array" <- w262
                n129 = Unbundle By Name(w259) -> ("COM Port"=w258:refnum<visa-resource-name>, "AG34970"=w257:refnum<visa-resource-name>)
                n130 = String Length(string=w265) -> (length=w269:i32)
                n131 = call "Agilent Scan EZ Temperature.vi"("VISA Resource Name"=w257, "Control"=enum16{"Initialize", "Read", "Experiment"}."Initialize", "Channel Input"=w265, "error in (no error)"=w271) -> ("error out"=w260:errorcluster)  [unwired: 8 in, 3 out]
                n132 = Greater Than 0?(x=w269) -> (x > 0?=w266:bool)
                "Use Agilent?" <- w266
                n133 = local read "Calibration File Array"() -> (w244:dbl[][])
                n134 = local read "GEA2 HyperData"() -> (w245:bool)
                n135 = Select(t=10, s=w245, f=1) -> (s? t:f=w249:i32)
                n136 = call "HEWH Serial Data Read.vi"("Serial Port Ref"=w258, "GEA2 HyperData"=w245, "Retries"=w249, "Serial Port Available?"=w242, "error in (no error)"=w260) -> ("Serial Read OK"=w243:bool, "Read String"=w267:string, "error out"=w248:errorcluster)  [unwired: 7 in, 1 out]
                "Serial Data In" <- w267
                n137 = control-ref of="Tank Display"() -> (w268:refnum<vi>)
                n138 = Compound Arithmetic op=AND(w242, invert w243) -> (w241:bool)
                n139 = call "Error Bool Add Message.vi"("Error?"=w241, "Message"="No Serial Data", "Error In"=w248) -> ("Error Out"=w247:errorcluster)  [unwired: 12 in]
                n140 = call "Gather Test Data - Heatup Test new.vi"("Agilent Scan List"=w265, "Semiphore"=w264, "Equipment"=w259, "Tank Display Ref"=w268, "Agilent?"=w266, "Calibration Coefficients"=w244, "error in (no error)"=w247, "Serial Data In"=w267, "Agilent Label Array"=w262) -> ("Output Data"=w253:string[][], "POWER"=w261:T3, "Voltage"=→"Voltage":dbl, "error out"=w256:errorcluster)  [unwired: 1 in, 2 out]
                n141 = local write "Current Log Data"(w253) -> ()
                n142 = local write "POWER"(w261) -> ()
                n143 = call-poly <vilib>:"Write To Spreadsheet File.vi"("delimiter (\\t)"="," ("delimiter (\\t)"), "append to file? (new file:F)"=TRUE, "2D data"=w253, "file path (dialog if empty)"=w252) -> ()  [unwired: 4 in, 1 out]
              }
              frame Error {
              }
            }
          }
          frame #3 {
            n144 = case shown="No Error" w274 {
              selector: w274 -> [_ w287]
              tunnel: [w280 w287] -> w276
              tunnel: w275 -> [w279 _]
              tunnel: w274 -> [w278 _]
              tunnel: w273 -> [w277 _]
              frame No Error {
                w281 = T21 [enum."Computation Start", enum."Reset Computation"] items=["Computation Start", "Computation stop", "Reset Computation", "Clear Computation"]
                # "Reset and restart computation of gallons."
                n145 = for {
                  tunnel: w281 -> [w284] mode=indexing
                  shift-right: [w285] -> w280
                  shift-left: w278 -> [w286]
                  tunnel: w279 -> [w283]
                  tunnel: w277 -> [w282]
                  n146 = call "YKMW100 Computation Control.vi"("VISA session"=w282, "Semiphore"=w283, "Mode"=w284, "error in (no error)"=w286) -> ("error out"=w285:errorcluster)  [unwired: 10 in, 1 out]
                }
              }
              frame Error {
              }
            }
          }
        }
        n147 = case shown="Error" w151 {
          selector: w151 -> [w299 w302]
          tunnel: [w298 string[] ["Finish"] ("States")] -> w164
          tunnel: [w299 w302] -> w163
          tunnel: w165 -> [w298 _]
          tunnel: [w297 w300] -> w159
          tunnel: w152 -> [w297 w300]
          tunnel: w149 -> [w288 _]
          frame No Error {
            w295 = ","
            w296 = TRUE ("Init Complete")
            n148 = local read "Computer Name"() -> (w294:string)
            n149 = local read "LAN IP Address"() -> (w290:string)
            n150 = local read "Ver."() -> (w293:string)
            n151 = property class="App"() -> ("App.Name"=w291:string)  [unwired: 2 in, 2 out]
            n152 = property on="Init Complete" class="Bool (strict)"("Val(Sgnl)"=w296) -> ()  [unwired: 2 in, 2 out]
            n153 = Concatenate Strings(w290, w295, w294, w295, w291, w295, w293, w295, "Started." ("string"), w295, w288) -> (w289:string)
            n154 = call "Save Time to File.vi"("String"=w289) -> ()  [unwired: 13 in, 2 out]
            "Init Complete" <- w296
          }
          frame Error {
          }
        }
      }
      frame "Wait for Purge" {
        # "wait for purge condition:\npower is off or...\nend of time is near or...\npurge condition tc > purge temp limit \nnote temp limit different between first and subsequent runs."
        n155 = local read "Purge Guard Time(s)"() -> (→"Purge Guard Time":dbl)
        n156 = local read "Purge0 Condition TC"() -> (→"Purge Condition TC":enum16{"TC1", "TC2", "TC3", "TC4", "TC5", "TC6"})
        n157 = local read "PurgreTempLimit"() -> (→"PurgreTempLimit":dbl)
        n158 = local read "Purgre0TempLim"() -> (→"Purgre0TempLim":dbl)
        n159 = local read "DrawCount"() -> (→"DrawCount":i32)
        n160 = property on="Monitoring Temps Chart" class="WFChart (strict)"(error in=w317, "History Data"=T8 []) -> (error out=w316:errorcluster)  [unwired: 1 in, 1 out]
        n161 = while {
          tunnel: w330 -> [w347]
          shift-right: [w345] -> w325
          shift-left: w316 -> [w344]
          tunnel: w329 -> [w346]
          tunnel: "Purge Guard Time(s)" -> [w340]
          i -> [w342]
          stop <- w341 stop-if-true
          # "stop waiting, on:\nerror gathering data,\ntemp limit reached,\nat end, use guard time,\nstop button"
          # "dont use\nserial for \nnow"
          n162 = local read "T1"() -> (w343:u32)
          n163 = Wait (ms)(milliseconds to wait=w343) -> ()  [unwired: 1 out]
          n164 = case shown="False" FALSE {
            tunnel: w347 -> [w399 w458]
            tunnel: w346 -> [w392 w454]
            tunnel: [w391 w452] -> w345
            tunnel: w344 -> [w390 w451]
            tunnel: w342 -> [w375 w440]
            tunnel: [w374 w414] -> w341
            tunnel: w340 -> [w369 w434]
            tunnel: "Skip Waiting for Temp" -> [w364 w433]
            tunnel: [w356 w415] -> w337
            frame True {
              n165 = local read "End Time(s)"() -> (w381:dbl)
              n166 = local read "Current Log Data"() -> (w359:string[][])
              n167 = local read "t*=0"() -> (w382:dbl)
              n168 = control-ref of="Tank Display"() -> (w361:refnum<vi>)
              n169 = call "E-Time.vi"("error in (no error)"=w390) -> ("error out"=w389:errorcluster, "Elapsed Time (sec)"=w383:dbl)  [unwired: 8 in, 1 out]
              n170 = Subtract(x=w383, y=w382) -> (x-y=w380:dbl)
              n171 = local read "Calibration File Array"() -> (w350:dbl[][])
              n172 = local read "Use Agilent?"() -> (w355:bool)
              n173 = Subtract(x=w381, y=w380) -> (x-y=w379:dbl)
              n174 = local read "Chanel List"() -> (w360:string)
              n175 = local read "Serial Data In"() -> (w353:string)
              n176 = local read "Label Array"() -> (w352:string[])
              n177 = Less?(x=w379, y=w369) -> (x < y?=w372:bool)
              n178 = call "Array_Search_For_Num.vi"("N Rows of Data"=w359, "Title?"="SetPoint") -> ("number"=w366:dbl)  [unwired: 12 in, 1 out]
              "SetPoint" <- w366
              n179 = call "Array_Search_For_Num.vi"("N Rows of Data"=w359, "Title?"="T2(TankSensor)") -> ("number"=w363:dbl)  [unwired: 12 in, 1 out]
              "T2(TankSensor)" <- w363
              n180 = Subtract(x=w366, y=w363) -> (x-y=w365:dbl)
              n181 = call "Gather Test Data - Heatup Test new.vi"("Agilent Scan List"=w360, "Semiphore"=w399, "Equipment"=w392, "Tank Display Ref"=w361, "Agilent?"=w355, "Calibration Coefficients"=w350, "error in (no error)"=w389, "Serial Data In"=w353, "Agilent Label Array"=w352) -> ("Tc Tree"=w387:dbl[], "Output Data"=w378:string[][], "POWER"=w351:T3, "Voltage"=w354:dbl, "error out"=w391:errorcluster)  [unwired: 1 in, 1 out]
              "Tcs 1-6" <- w387
              n182 = local write "Voltage"(w354) -> ()
              n183 = Array To Cluster(array=w387) -> (cluster=w397:T22)
              n184 = local write "POWER"(w351) -> ()
              n185 = local read "DrawCount"() -> (w371:i32)
              n186 = Build Array(w397) -> (→"Monitoring Temps Chart":T8)
              n187 = Number To Decimal String(number=w375) -> (decimal integer string=w393:string)  [unwired: 1 in]
              n188 = Less?(x=w365, y="T2_Threshold") -> (x < y?=w358:bool)
              n189 = Number To Fractional String(number=w363) -> (F-format string=w385:string)  [unwired: 3 in]
              n190 = Equal To 0?(x=w375) -> (x = 0?=w376:bool)
              n191 = Greater Than 0?(x=w371) -> (x > 0?=w370:bool)
              n192 = Greater Than 0?(x=w365) -> (x > 0?=w388:bool)
              n193 = Concatenate Strings("Wating for Purge Condition. T2 Tank > Threshold. T2(tank)= " ("string"), w385, ". " ("string"), w393, "Readings" ("string")) -> (w394:string)
              n194 = And(x=w388, y=w364) -> (x .and. y?=w356:bool)
              n195 = call "String_in_Reference.vi"("String"=w394) -> ()  [unwired: 18 in, 1 out]
              n196 = And(x=w372, y=w370) -> (x .and. y?=w373:bool)
              n197 = Unbundle By Name(w391) -> ("status"=w398:bool)
              n198 = local read "Stop Test"() -> (w357:bool)
              n199 = Compound Arithmetic op=OR(w398, w358, w356, w373, w357) -> (w374:bool)
              n200 = Compound Arithmetic op=OR(w376, w374) -> (w377:bool)
              n201 = case shown="True" w377 {
                tunnel: w378 -> [_ w401]
                frame False {
                }
                frame True {
                  n202 = Index Array(array=w401, index (row)=1) -> (element=w400:string[])  [unwired: 1 in]
                  n203 = local read "FileName"() -> (w405:path)
                  n204 = call-poly <vilib>:"Write To Spreadsheet File.vi"("delimiter (\\t)"="," ("delimiter (\\t)"), "append to file? (new file:F)"=TRUE, "1D data"=w400, "file path (dialog if empty)"=w405) -> ()  [unwired: 4 in, 1 out]
                }
              }
            }
            frame False {
              # "err"
              n205 = local read "Serial Data In"() -> (w410:string)
              n206 = local read "DrawCount"() -> (w437:i32)
              n207 = local read "Chanel List"() -> (w442:string)
              n208 = local read "t*=0"() -> (w446:dbl)
              n209 = call "E-Time.vi"("error in (no error)"=w451) -> ("error out"=w450:errorcluster, "Elapsed Time (sec)"=w447:dbl)  [unwired: 8 in, 1 out]
              n210 = local read "Use Agilent?"() -> (w412:bool)
              n211 = local read "Label Array"() -> (w409:string[])
              n212 = Greater Than 0?(x=w437) -> (x > 0?=w407:bool)
              n213 = case shown="True" w407 {
                tunnel: ["Purge0 Condition TC" "Purge Condition TC"] -> w408
                frame False {
                }
                frame True {
                }
              }
              n214 = local read "Calibration File Array"() -> (w406:dbl[][])
              n215 = local read "End Time(s)"() -> (w445:dbl)
              n216 = Increment(x=w408) -> (x+1=w424:enum16{"TC1", "TC2", "TC3", "TC4", "TC5", "TC6"})
              n217 = Subtract(x=w447, y=w446) -> (x-y=w444:dbl)
              n218 = Select(t="PurgreTempLimit", s=w407, f="Purgre0TempLim") -> (s? t:f=w426:dbl)
              n219 = control-ref of="Tank Display"() -> (w453:refnum<vi>)
              n220 = Number To Decimal String(number=w424) -> (decimal integer string=w431:string)  [unwired: 1 in]
              n221 = Subtract(x=w445, y=w444) -> (x-y=w443:dbl)
              n222 = Less?(x=w443, y=w434) -> (x < y?=w438:bool)
              n223 = call "Gather Test Data - Heatup Test new.vi"("Agilent Scan List"=w442, "Semiphore"=w458, "Equipment"=w454, "Tank Display Ref"=w453, "Agilent?"=w412, "Calibration Coefficients"=w406, "error in (no error)"=w450, "Serial Data In"=w410, "Agilent Label Array"=w409) -> ("Tc Tree"=w435:dbl[], "Output Data"=w416:string[][], "POWER"=w429:T3, "Voltage"=w411:dbl, "error out"=w452:errorcluster)  [unwired: 1 in, 1 out]
              n224 = local write "POWER"(w429) -> ()
              n225 = local write "Tcs 1-6"(w435) -> ()
              n226 = Index Array(array=w435, index=w408) -> (element=w425:dbl)
              n227 = Number To Decimal String(number=w426) -> (decimal integer string=w448:string)  [unwired: 1 in]
              n228 = Number To Decimal String(number=w440) -> (decimal integer string=w420:string)  [unwired: 1 in]
              n229 = Greater Than 0?(x=w425) -> (x > 0?=w449:bool)
              n230 = Array To Cluster(array=w435) -> (cluster=w455:T22)
              n231 = local write "Current Log Data"(w416) -> ()
              n232 = Greater?(x=w425, y=w426) -> (0:w457:bool)
              n233 = Concatenate Strings(" Purge Condition. T" ("string"), w431, " > " ("string"), w448) -> (w418:string)
              n234 = Equal To 0?(x=w440) -> (x = 0?=w423:bool)
              n235 = And(x=w449, y=w433) -> (x .and. y?=w415:bool)
              n236 = local write "Voltage"(w411) -> ()
              n237 = Build Array(w455) -> (w436:T8)
              n238 = Concatenate Strings(". " ("string"), w420, "Readings" ("string")) -> (w419:string)
              n239 = local write "Monitoring Temps Chart"(w436) -> ()
              n240 = Unbundle By Name(w452) -> ("status"=w456:bool)
              n241 = Concatenate Strings(w418, w419) -> (w417:string)
              n242 = call "String_in_Reference.vi"("String"=w417) -> ()  [unwired: 18 in, 1 out]
              n243 = And(x=w438, y=w407) -> (x .and. y?=w439:bool)
              n244 = local read "Stop Test"() -> (w413:bool)
              n245 = case shown="True" w423 {
                tunnel: w418 -> [_ w461]
                frame False {
                }
                frame True {
                  n246 = local read "FileName"() -> (w462:path)
                  n247 = call "Log String to Spreadsheet.vi"("String"=w461, "FileName"=w462) -> ()  [unwired: 9 in, 1 out]
                }
              }
              n248 = Compound Arithmetic op=OR(w456, w457, w415, w439, w413) -> (w414:bool)
              n249 = Compound Arithmetic op=OR(w423, w414) -> (w441:bool)
              n250 = case shown="True" w441 {
                tunnel: w416 -> [_ w464]
                frame False {
                }
                frame True {
                  # "log at beg. and end."
                  n251 = Index Array(array=w464, index (row)=1) -> (element=w463:string[])  [unwired: 1 in]
                  n252 = local read "FileName"() -> (w468:path)
                  n253 = call-poly <vilib>:"Write To Spreadsheet File.vi"("delimiter (\\t)"="," ("delimiter (\\t)"), "append to file? (new file:F)"=TRUE, "1D data"=w463, "file path (dialog if empty)"=w468) -> ()  [unwired: 4 in, 1 out]
                }
              }
            }
          }
          n254 = case shown="True" w337 {
            frame False {
            }
            frame True {
              n255 = local read "FileName"() -> (w349:path)
              n256 = call "Log String to Spreadsheet.vi"("String"="Skipped waiting", "FileName"=w349) -> ()  [unwired: 9 in, 1 out]
            }
          }
        }
        n257 = case shown="Error" w325 {
          selector: w325 -> [w333 w336]
          tunnel: [w334 string[] ["Finish"] ("States")] -> w327
          tunnel: w328 -> [w334 _]
          tunnel: [w333 w336] -> w326
          frame No Error {
            # "Press it each time."
            n258 = local write "Skip Waiting for Temp"(FALSE ("Skip Waiting for Temp")) -> ()
          }
          frame Error {
          }
        }
      }
      frame "Purge" {
        # "Used in Reference in Purge Routine."
        # "Purge Ends at 1 GPM now."
        n259 = local read "RTD 2 Downspout offset"() -> (w476:dbl)
        n260 = local read "Temp Band(+/- F)"() -> (w481:dbl)
        n261 = local read "Flow rate setting"() -> (w480:dbl)
        n262 = local read "Degree Setting"() -> (w477:dbl)
        n263 = Subtract(x=w477, y=w476) -> (x-y=w478:dbl)
        n264 = case shown="False" "Skip Purge" {
          tunnel: w481 -> [w496 _]
          tunnel: w480 -> [w494 _]
          tunnel: w479 -> [w493 w499]
          tunnel: w478 -> [w490 _]
          tunnel: [w489 w499] -> w469
          tunnel: w472 -> [w488 _]
          tunnel: w471 -> [w487 _]
          frame False {
            n265 = control-ref of="Downspount Flow"() -> (w498:refnum<vi>)
            n266 = control-ref of="Purge Temperature"() -> (w492:refnum<vi>)
            n267 = call "Purge Water Sequence SM.vi"("Degree Setting"=w490, "Equipment"=w488, "Semiphore"=w487, "Flow rate setting"=w494, "Temp Band(+/- F)"=w496, "Error In"=w493, "Flow Chart Ref"=w498, "Temp Chart Ref"=w492) -> ("Downspout Flow"=→"Downspout Flow":dbl, "Downspout Temp"=→"Downspout Temp":dbl, "Flow rate setting out"=→"Flow rate Adj":dbl, "Temp Setting Out"=→"Temp Adj":dbl, "Error Out"=w489:errorcluster)  [unwired: 2 in, 1 out]
          }
          frame True {
          }
        }
        n268 = flat-sequence {
          tunnel: [w506] -> w475
          tunnel: w469 -> [w505]
          frame #0 {
            w508 = "PurgeEnds" ("string")
            n269 = local read "FileName"() -> (w507:path)
            n270 = call "String_in_Reference.vi"("String"=w508) -> ()  [unwired: 18 in, 1 out]
            n271 = call "Log String to Spreadsheet.vi"("String"=w508, "error in (no error)"=w505, "FileName"=w507) -> ("error out"=w506:errorcluster)  [unwired: 8 in]
          }
        }
        n272 = Unbundle By Name(w475) -> ("source"=w474:string)
        n273 = case shown="\"True\", Default" w474 {
          selector: w474 -> [_ w502]
          tunnel: w475 -> [w500 w503]
          tunnel: [w500 w501] -> w473
          frame "" {
          }
          frame "True", Default {
            # "Temp not stable case may\njust posts this warning."
            n274 = local read "FileName"() -> (w504:path)
            n275 = call "Log String to Spreadsheet.vi"("String"=w502, "error in (no error)"=w503, "FileName"=w504) -> ("error out"=w501:errorcluster)  [unwired: 8 in]
          }
        }
        n276 = case shown="No Error" w473 {
          selector: w473 -> [w509 w512]
          tunnel: [w510 string[] ["Finish"] ("States")] -> w485
          tunnel: w483 -> [w510 _]
          tunnel: [w509 w512] -> w484
          frame No Error {
          }
          frame Error {
          }
        }
      }
      frame "Wait for Cutout" {
        # "If Ave Temp not in range, display error."
        # "The second time through, before the start of the test, make sure the temp is in range."
        n277 = while {
          tunnel: w518 -> [w551]
          shift-right: [w550] -> w517
          shift-left: w515 -> [w536]
          tunnel: ["Skip Waiting for Cutout"] -> w514
          tunnel: [w541] -> w513
          i -> [w544]
          stop <- w547 continue-if-true
          n278 = local read "T1"() -> (w534:u32)
          n279 = call "Delay mS.vi"("Error In"=w536, "milliseconds to wait"=w534) -> ("Error Out"=w535:errorcluster)  [unwired: 13 in]
          n280 = local read "Calibration File Array"() -> (w531:dbl[][])
          n281 = local read "Use Agilent?"() -> (w537:bool)
          n282 = local read "Serial Data In"() -> (w539:string)
          n283 = local read "Label Array"() -> (w538:string[])
          n284 = control-ref of="Tank Display"() -> (w552:refnum<vi>)
          n285 = local read "Chanel List"() -> (w549:string)
          n286 = local read "Equipment"() -> (w553:T6)
          n287 = call "Gather Test Data - Heatup Test new.vi"("Agilent Scan List"=w549, "Semiphore"=w551, "Equipment"=w553, "Tank Display Ref"=w552, "Agilent?"=w537, "Calibration Coefficients"=w531, "error in (no error)"=w535, "Serial Data In"=w539, "Agilent Label Array"=w538) -> ("Tc Tree"=w541:dbl[], "Output Data"=w548:string[][], "POWER"=w533:T3, "Voltage"=w540:dbl, "error out"=w550:errorcluster)  [unwired: 1 in, 1 out]
          n288 = local write "Current Log Data"(w548) -> ()
          n289 = local write "POWER"(w533) -> ()
          n290 = local write "Voltage"(w540) -> ()
          n291 = call "HEWH Heat Elements Interpretation.vi"("POWER"=w533) -> ("Comp or HE No Error"=w532:bool)  [unwired: 11 in, 3 out]
          n292 = local read "Stop Test"() -> (w543:bool)
          n293 = Number To Decimal String(number=w544) -> (decimal integer string=w554:string)  [unwired: 1 in]
          n294 = Unbundle By Name(w550) -> ("status"=w558:bool)
          n295 = Equal To 0?(x=w544) -> (x = 0?=w545:bool)
          n296 = Compound Arithmetic op=AND(invert w558, w532, invert "Skip Waiting for Cutout", invert w543) -> (w547:bool)
          n297 = Compound Arithmetic op=OR(w545, invert w547) -> (w546:bool)
          n298 = Concatenate Strings("WAIT FOR CUTOUT.  " ("String"), w554, " checks." ("string")) -> (w556:string)
          n299 = case shown="True" w546 {
            tunnel: w548 -> [_ w561]
            frame False {
            }
            frame True {
              n300 = Index Array(array=w561, index (row)=1) -> (element=w564:string[])  [unwired: 1 in]
              n301 = local read "FileName"() -> (w560:path)
              n302 = call-poly <vilib>:"Write To Spreadsheet File.vi"("delimiter (\\t)"="," ("delimiter (\\t)"), "append to file? (new file:F)"=TRUE, "1D data"=w564, "file path (dialog if empty)"=w560) -> ()  [unwired: 4 in, 1 out]
            }
          }
          n303 = call "String_in_Reference.vi"("String"=w556) -> ()  [unwired: 18 in, 1 out]
        }
        n304 = case shown="False" w514 {
          tunnel: w517 -> [w524 w528]
          tunnel: [w523 w527] -> w516
          frame True {
            n305 = local read "FileName"() -> (w526:path)
            n306 = call "Log String to Spreadsheet.vi"("String"="Skipped waiting for Cutout", "error in (no error)"=w524, "FileName"=w526) -> ("error out"=w523:errorcluster)  [unwired: 8 in]
          }
          frame False {
            n307 = local read "FileName"() -> (w530:path)
            n308 = call "Log String to Spreadsheet.vi"("String"="Cutout", "error in (no error)"=w528, "FileName"=w530) -> ("error out"=w527:errorcluster)  [unwired: 8 in]
          }
        }
        n309 = case shown="No Error" w516 {
          selector: w516 -> [w577 w595]
          tunnel: [w575 string[] ["Finish"] ("States")] -> w522
          tunnel: w520 -> [w570 _]
          tunnel: [w576 w594] -> w521
          tunnel: w513 -> [w574 _]
          frame No Error {
            # "Press Each Time"
            n310 = local read "DrawCount"() -> (w572:i32)
            n311 = local write "Skip Waiting for Cutout"(FALSE ("Skip Waiting for Cutout")) -> ()
            n312 = Index Array(array=w570, index=0) -> (element=w568:string)
            n313 = Equal?(x=w572, y=0) -> (x = y?=w566:bool)
            n314 = Equal?(x=w568, y="Wait for Temp Decl") -> (x = y?=w567:bool)
            n315 = And(x=w567, y=w566) -> (x .and. y?=w565:bool)
            n316 = case shown="True" w565 {
              tunnel: w574 -> [_ w589]
              tunnel: [w580 w584] -> w575
              tunnel: w570 -> [w580 w583]
              tunnel: [w579 w582] -> w576
              tunnel: w577 -> [w579 w581]
              frame False {
              }
              frame True {
                n317 = call-poly <vilib>:"Mean.vi"("X"=w589) -> ("mean"=w588:dbl)  [unwired: 1 out]
                "Ave Tank Temp" <- w588
                n318 = In Range and Coerce(upper limit="mean tank upper lim", x=w588, lower limit="meant tank lower lim") -> (In Range?=w585:bool)  [unwired: 1 out]
                n319 = case shown="True" w585 {
                  tunnel: [string[] ["Finish"] w593] -> w584
                  tunnel: w583 -> [_ w593]
                  tunnel: [errorcluster {"status"=TRUE, "code"=-7101, "source"="Check Tank Temp Setting"} ("error IO") w592] -> w582
                  tunnel: w581 -> [_ w592]
                  frame False {
                  }
                  frame True {
                  }
                }
              }
            }
          }
          frame Error {
            n320 = local read "FileName"() -> (w596:path)
            n321 = call "Log String to Spreadsheet.vi"("String"="Error", "error in (no error)"=w595, "FileName"=w596) -> ("error out"=w594:errorcluster)  [unwired: 8 in]
          }
        }
      }
      frame "Wait for Temp Decl" {
        n322 = local read "FileName"() -> (w607:path)
        n323 = Number To Fractional String(number="Temp Decline Hystersis") -> (F-format string=w603:string)  [unwired: 3 in]
        n324 = Concatenate Strings("Record each new Tave maximum.  Wating for Ave temp to decl by   " ("string"), w603, "degrees F." ("string")) -> (w600:string)
        n325 = call "Log String to Spreadsheet.vi"("String"=w600, "error in (no error)"=w602, "FileName"=w607) -> ("error out"=w601:errorcluster)  [unwired: 8 in]
        n326 = while {
          tunnel: w612 -> [w664]
          shift-right: [w648] -> w610
          shift-left: w601 -> [w663]
          tunnel: w611 -> [w652]
          shift-right: [w642] -> w608
          shift-left: 0.0 ("T_Ave_Max") -> [w641]
          tunnel: "Temp Decline Hystersis" -> [w637]
          tunnel: ["Skip Waiting for Temp 3"] -> w599
          i -> [w650]
          stop <- w638 stop-if-true
          n327 = local read "Serial Data In"() -> (w633:string)
          n328 = local read "Use Agilent?"() -> (w631:bool)
          n329 = local read "Label Array"() -> (w632:string[])
          n330 = local read "Calibration File Array"() -> (w630:dbl[][])
          n331 = local read "Chanel List"() -> (w647:string)
          n332 = control-ref of="Tank Display"() -> (w651:refnum<vi>)
          n333 = Number To Decimal String(number=w650) -> (decimal integer string=w655:string)  [unwired: 1 in]
          n334 = call "Gather Test Data - Heatup Test new.vi"("Agilent Scan List"=w647, "Semiphore"=w664, "Equipment"=w652, "Tank Display Ref"=w651, "Agilent?"=w631, "Calibration Coefficients"=w630, "error in (no error)"=w663, "Serial Data In"=w633, "Agilent Label Array"=w632) -> ("Tc Tree"=w658:dbl[], "Output Data"=w644:string[][], "POWER"=w643:T3, "Voltage"=w634:dbl, "error out"=w648:errorcluster)  [unwired: 1 in, 1 out]
          n335 = local write "Voltage"(w634) -> ()
          n336 = local write "POWER"(w643) -> ()
          n337 = call-poly <vilib>:"Mean.vi"("X"=w658) -> ("mean"=w645:dbl)  [unwired: 1 out]
          "T_Ave" <- w645
          n338 = Max & Min(x=w641, y=w645) -> (max(x,y)=w642:dbl)  [unwired: 1 out]
          "T_Ave_Max" <- w642
          n339 = Build Array (concatenate)(w658, w645) -> (w653:dbl[])
          "Tcs 1-6, Ave. 3" <- w653
          n340 = Concatenate Strings("Wating for Ave temp to decl.  " ("string"), w655, "Readings" ("string")) -> (w656:string)
          n341 = local write "Current Log Data"(w644) -> ()
          n342 = call "String_in_Reference.vi"("String"=w656) -> ()  [unwired: 18 in, 1 out]
          n343 = Array To Cluster(array=w653) -> (cluster=w660:T23)
          n344 = Subtract(x=w642, y=w645) -> (x-y=w646:dbl)
          n345 = Greater?(x=w642, y=w641) -> (0:w640:bool)
          n346 = Build Array(w660) -> (→"Temps Chart 2":T9)
          n347 = local read "Stop Test"() -> (w636:bool)
          n348 = Greater Or Equal?(x=w646, y=w637) -> (x >= y?=w662:bool)
          n349 = Unbundle By Name(w648) -> ("status"=w661:bool)
          n350 = local read "T1"() -> (w649:u32)
          n351 = Compound Arithmetic op=OR(w661, w662, "Skip Waiting for Temp 3", w636) -> (w638:bool)
          n352 = Compound Arithmetic op=OR(w640, w638) -> (w639:bool)
          n353 = case shown="True" w639 {
            tunnel: w644 -> [_ w665]
            frame False {
            }
            frame True {
              n354 = Index Array(array=w665, index (row)=1) -> (element=w666:string[])  [unwired: 1 in]
              n355 = local read "FileName"() -> (w670:path)
              n356 = call-poly <vilib>:"Write To Spreadsheet File.vi"("delimiter (\\t)"="," ("delimiter (\\t)"), "append to file? (new file:F)"=TRUE, "1D data"=w666, "file path (dialog if empty)"=w670) -> ()  [unwired: 4 in, 1 out]
            }
          }
          n357 = Wait (ms)(milliseconds to wait=w649) -> ()  [unwired: 1 out]
        }
        n358 = case shown="True" w599 {
          tunnel: [w623 w627] -> w613
          tunnel: w610 -> [w622 w628]
          tunnel: w608 -> [w619 _]
          frame False {
            n359 = Number To Fractional String(number=w619) -> (F-format string=w621:string)  [unwired: 3 in]
            n360 = local read "FileName"() -> (w624:path)
            n361 = Concatenate Strings("Ave Temp Declined. Max Ave Tank Temp = " ("String"), w621) -> (w620:string)
            n362 = call "Log String to Spreadsheet.vi"("String"=w620, "error in (no error)"=w622, "FileName"=w624) -> ("error out"=w623:errorcluster)  [unwired: 8 in]
          }
          frame True {
            n363 = local write "Skip Waiting for Temp 3"(FALSE ("Skip Waiting for Temp 3")) -> ()
            n364 = local read "FileName"() -> (w629:path)
            n365 = call "Log String to Spreadsheet.vi"("String"="Skipped Waiting for Temp Decl", "error in (no error)"=w628, "FileName"=w629) -> ("error out"=w627:errorcluster)  [unwired: 8 in]
          }
        }
        n366 = case shown="No Error" w613 {
          selector: w613 -> [w671 w675]
          tunnel: [w672 string[] ["Finish"] ("States")] -> w617
          tunnel: w615 -> [w672 _]
          tunnel: [w671 w674] -> w616
          frame No Error {
          }
          frame Error {
            n367 = local read "FileName"() -> (w676:path)
            n368 = call "Log String to Spreadsheet.vi"("String"="Error", "error in (no error)"=w675, "FileName"=w676) -> ("error out"=w674:errorcluster)  [unwired: 8 in]
          }
        }
      }
      frame "Init Draw" {
        # "Make sure stop button not depressed."
        # "Fail Condition Before start of a Draw."
        n369 = local read "Special Last Draw"() -> (w679:bool)
        n370 = case shown="False" w679 {
          tunnel: w683 -> [w699 w720]
          tunnel: [w698 w724] -> w682
          tunnel: w681 -> [w697 w723]
          tunnel: [w710 TRUE] -> w678
          frame False {
            # "Init T*Max"
            n371 = local read "Serial Data In"() -> (w692:string)
            n372 = local read "Use Agilent?"() -> (w690:bool)
            n373 = local read "Calibration File Array"() -> (w689:dbl[][])
            n374 = local read "Label Array"() -> (w691:string[])
            n375 = control-ref of="Tank Display"() -> (w700:refnum<vi>)
            n376 = local read "Chanel List"() -> (w708:string)
            n377 = local read "Equipment"() -> (w701:T6)
            n378 = call "Gather Test Data - Heatup Test new.vi"("Agilent Scan List"=w708, "Semiphore"=w697, "Equipment"=w701, "Tank Display Ref"=w700, "Agilent?"=w690, "Calibration Coefficients"=w689, "error in (no error)"=w699, "Serial Data In"=w692, "Agilent Label Array"=w691) -> ("Tc Tree"=w695:dbl[], "Output Data"=w706:string[][], "POWER"=w709:T3, "Voltage"=w693:dbl, "error out"=w698:errorcluster)  [unwired: 1 in, 1 out]
            n379 = local write "Current Log Data"(w706) -> ()
            n380 = local read "FileName"() -> (w702:path)
            n381 = Index Array(array=w706, index (row)=1) -> (element=w707:string[])  [unwired: 1 in]
            n382 = Index Array(array=w695, index=0) -> (element=w696:dbl)
            n383 = call-poly <vilib>:"Write To Spreadsheet File.vi"("delimiter (\\t)"="," ("delimiter (\\t)"), "append to file? (new file:F)"=TRUE, "1D data"=w707, "file path (dialog if empty)"=w702) -> ()  [unwired: 4 in, 1 out]
            n384 = local write "Voltage"(w693) -> ()
            n385 = local write "POWER"(w709) -> ()
            n386 = In Range and Coerce(upper limit="Tc1 UL", x=w696, lower limit="Tc1 LL") -> (In Range?=w710:bool)  [unwired: 1 out]
          }
          frame True {
            n387 = local read "Use Agilent?"() -> (w717:bool)
            n388 = local read "Serial Data In"() -> (w715:string)
            n389 = local read "FileName"() -> (w721:path)
            n390 = local read "Label Array"() -> (w714:string[])
            n391 = call "Log String to Spreadsheet.vi"("String"="Start Last Draw.", "error in (no error)"=w720, "FileName"=w721) -> ("error out"=w719:errorcluster)  [unwired: 8 in]
            n392 = local read "Chanel List"() -> (w733:string)
            n393 = control-ref of="Tank Display"() -> (w725:refnum<vi>)
            n394 = local read "Calibration File Array"() -> (w713:dbl[][])
            n395 = local read "Equipment"() -> (w726:T6)
            n396 = call "Gather Test Data - Heatup Test new.vi"("Agilent Scan List"=w733, "Semiphore"=w723, "Equipment"=w726, "Tank Display Ref"=w725, "Agilent?"=w717, "Calibration Coefficients"=w713, "error in (no error)"=w719, "Serial Data In"=w715, "Agilent Label Array"=w714) -> ("Output Data"=w731:string[][], "POWER"=w734:T3, "Voltage"=w716:dbl, "error out"=w724:errorcluster)  [unwired: 1 in, 2 out]
            n397 = local write "Current Log Data"(w731) -> ()
            n398 = local write "Voltage"(w716) -> ()
            n399 = local write "POWER"(w734) -> ()
            n400 = Index Array(array=w731, index (row)=1) -> (element=w732:string[])  [unwired: 1 in]
            n401 = local read "FileName"() -> (w727:path)
            n402 = call-poly <vilib>:"Write To Spreadsheet File.vi"("delimiter (\\t)"="," ("delimiter (\\t)"), "append to file? (new file:F)"=TRUE, "1D data"=w732, "file path (dialog if empty)"=w727) -> ()  [unwired: 4 in, 1 out]
          }
        }
        n403 = call "String_in_Reference.vi"("String"="Init Draw") -> ()  [unwired: 18 in, 1 out]
        n404 = case shown="True" w678 {
          tunnel: [w735 w758] -> w685
          tunnel: w682 -> [_ w746]
          tunnel: w681 -> [_ w742]
          frame False {
            n405 = call "Error Bool Enumerator.vi"("Error Enum"=HEWH_Error_Enumeration."Init Draw: TC_1 Out of Range") -> ("Error Out"=w735:errorcluster)  [unwired: 8 in]
            n406 = Unbundle By Name(w735) -> ("source"=w737:string)
            n407 = local read "FileName"() -> (w738:path)
            n408 = call "Log String to Spreadsheet.vi"("String"=w737, "FileName"=w738) -> ()  [unwired: 9 in, 1 out]
          }
          frame True {
            # "Anti Waterhamer"
            n409 = local read "Flow Adj Draw"() -> (w740:dbl)
            n410 = local read "MW100"() -> (w743:refnum<visa-resource-name>)
            n411 = local read "Stop Logging"() -> (w751:bool)
            n412 = local read "Stop Test"() -> (w750:bool)
            n413 = local read "Stop"() -> (w749:bool)
            n414 = call "Linear Interpolation GPM to Percent Open.vi"("Input (GPM,Percent)"=w740) -> ("Output (Percent,GPM)"=w739:dbl)  [unwired: 10 in]
            n415 = local read "DrawCount"() -> (w748:i32)
            n416 = Compound Arithmetic op=AND(invert w749, invert w751, invert w750) -> (w752:bool)
            n417 = call "Intellifaucet_Driver.vi"("VISA session"=w743, "Mode"=Intellfaucet_Mode."Adjust Flow", "Semiphore"=w742, "Percent Flow"=w739) -> ("VISA session out"=w744:refnum<visa-resource-name>)  [unwired: 10 in, 1 out]
            n418 = Not Equal To 0?(x=w748) -> (x != 0?=w747:bool)
            n419 = case shown="True" w752 {
              tunnel: [w765 w775] -> w745
              tunnel: w744 -> [w764 w771]
              tunnel: w742 -> [_ w769]
              tunnel: w746 -> [w765 w772]
              tunnel: w747 -> [_ w776]
              tunnel: [w764 w774] -> _
              frame False {
              }
              frame True {
                n420 = call "Solenoid Bank.vi"("VISA session"=w771, "Semiphore"=w769, "Drain Valve"=enum8{"OPEN", "CLOSE"}."CLOSE", "Output Valve"=enum8{"CLOSE", "OPEN"}."OPEN", "Input Valve"=enum8{"OPEN", "CLOSE"}."OPEN", "Error In"=w772) -> ("dup VISA session"=w770:refnum<visa-resource-name>, "Error Out"=w773:errorcluster)  [unwired: 8 in]
                n421 = call "HEWH Totalize Flow Control.vi"("VISA session"=w770, "Semiphore"=w769, "Totalize Flow"=w776, "error in (no error)"=w773) -> ("dup VISA session"=w774:refnum<visa-resource-name>, "error out"=w775:errorcluster)  [unwired: 10 in]
              }
            }
            n422 = Equal?(x=1, y=w748) -> (x = y?=w757:bool)
            n423 = call "E-Time.vi"("error in (no error)"=w745) -> ("error out"=w755:errorcluster, "Elapsed Time (sec)"=w753:dbl)  [unwired: 8 in, 1 out]
            "Current Draw Start Time" <- w753
            n424 = case shown="True" w757 {
              tunnel: w755 -> [w777 w779]
              tunnel: [w777 w784] -> w762
              tunnel: w753 -> [_ w778]
              frame False {
              }
              frame True {
                n425 = local write "t*=0"(w778) -> ()
                n426 = Number To Fractional String(number=w778) -> (F-format string=w781:string)  [unwired: 3 in]
                n427 = local read "FileName"() -> (w783:path)
                n428 = Concatenate Strings("t0*=", w781) -> (w780:string)
                n429 = call "Log String to Spreadsheet.vi"("String"=w780, "error in (no error)"=w779, "FileName"=w783) -> ("error out"=w784:errorcluster)  [unwired: 8 in]
              }
            }
            n430 = Number To Hexadecimal String(2:w748) -> (0:w759:string)  [unwired: 1 in]
            n431 = Concatenate Strings("DrawCount = " ("string"), w759, ".  Current Draw Start Time:" ("string")) -> (w761:string)
            n432 = local read "FileName"() -> (w763:path)
            n433 = call "Log String to Spreadsheet.vi"("String"=w761, "error in (no error)"=w762, "FileName"=w763) -> ("error out"=w758:errorcluster)  [unwired: 8 in]
          }
        }
        n434 = case shown="No Error" w685 {
          selector: w685 -> [w789 w797]
          tunnel: [w790 string[] ["Finish"] ("States")] -> w686
          tunnel: w687 -> [w790 _]
          tunnel: [w788 w797] -> w684
          frame No Error {
            # "To turn of 10 sec sampling."
            n435 = local read "Flow rate Adj"() -> (w787:dbl)
            n436 = local read "Temp Adj"() -> (w786:dbl)
            n437 = disable-structure shown="Enabled" {
              disable-tunnel: w789 -> [w792 w795]
              disable-tunnel: [w791 w795] -> w788
              frame Enabled {
                n438 = flat-sequence {
                  tunnel: [w794] -> w791
                  tunnel: w792 -> [w794]
                  frame #0 {
                    "Drawing" <- TRUE
                  }
                }
              }
              frame Disabled {
                # "FIXME put back for real app.!"
              }
            }
            n439 = local write "Temp Adj Draw"(w786) -> ()
            n440 = local write "Flow Adj Draw"(w787) -> ()
            "T*max" <- 0.0 ("T*max")
          }
          frame Error {
          }
        }
      }
      frame "Wait for Next Draw" {
        # "initiate successive draws\nwhen the applicable thermostat acts to reduce\nthe electrical input to the element located\nvertically highest in the storage tank."
        # "1. A draw is going at t-1 hr, complete\n2a. a draw is not going, immediately start and continue for at least 30 seconds\n2b.  If after 30 sec, T< last tmin, stop and discard measurements, else continue"
        n441 = local read "DrawCount"() -> (w799:i32)
        n442 = local read "End Time(s)"() -> (w802:dbl)
        n443 = local read "t*=0"() -> (w805:dbl)
        n444 = call "E-Time.vi"("error in (no error)"=w809) -> ("error out"=w808:errorcluster, "Elapsed Time (sec)"=w803:dbl)  [unwired: 8 in, 1 out]
        n445 = Subtract(x=w803, y=w805) -> (x-y=w804:dbl)
        n446 = Equal To 0?(x=w799) -> (x = 0?=w798:bool)
        n447 = Less?(x=w804, y=w802) -> (x < y?=w801:bool)
        n448 = Or(x=w801, y=w798) -> (x .or. y?=w800:bool)
        n449 = case shown="True" w800 {
          tunnel: w806 -> [_ w818]
          tunnel: [w813 w820] -> w811
          tunnel: w808 -> [w813 w815]
          tunnel: [string[] ["Finish"] ("States") w821] -> w807
          frame False {
            # "Time elapsed during last draw."
          }
          frame True {
            w816 = "Wait for Power decrease." ("string")
            # "in eheat use the compressor as signal to start next draw, otherwise upper element."
            n450 = local read "FileName"() -> (w817:path)
            n451 = call "String_in_Reference.vi"("String"=w816) -> ()  [unwired: 18 in, 1 out]
            n452 = call "Log String to Spreadsheet.vi"("String"=w816, "error in (no error)"=w815, "FileName"=w817) -> ("error out"=w814:errorcluster)  [unwired: 8 in]
            n453 = while {
              tunnel: w818 -> [w839]
              shift-right: [w858] -> w819
              shift-left: w814 -> [w840]
              tunnel: [w845] -> w822
              i -> [w836]
              stop <- w835 continue-if-true
              n454 = local read "T1"() -> (w853:u32)
              n455 = local read "Serial Data In"() -> (w831:string)
              n456 = local read "Chanel List"() -> (w844:string)
              n457 = local read "Label Array"() -> (w830:string[])
              n458 = control-ref of="Tank Display"() -> (w841:refnum<vi>)
              n459 = Wait (ms)(milliseconds to wait=w853) -> ()  [unwired: 1 out]
              n460 = local read "Calibration File Array"() -> (w823:dbl[][])
              n461 = local read "Mode"() -> (w827:T7)
              n462 = local read "Equipment"() -> (w842:T6)
              n463 = call "Gather Test Data - Heatup Test new.vi"("Agilent Scan List"=w844, "Semiphore"=w839, "Equipment"=w842, "Tank Display Ref"=w841, "Calibration Coefficients"=w823, "error in (no error)"=w840, "Serial Data In"=w831, "Agilent Label Array"=w830) -> ("Output Data"=w843:string[][], "POWER"=w826:T3, "Voltage"=w829:dbl, "error out"=w838:errorcluster)  [unwired: 2 in, 2 out]
              n464 = Number To Decimal String(number=w836) -> (decimal integer string=w854:string)  [unwired: 1 in]
              n465 = local write "Current Log Data"(w843) -> ()
              n466 = local write "Voltage"(w829) -> ()
              n467 = local write "POWER"(w826) -> ()
              n468 = call "HEWH Heat Elements Interpretation.vi"("POWER"=w826) -> ("UE and No Error"=w825:bool, "Com and No Error"=w824:bool)  [unwired: 11 in, 2 out]
              n469 = local read "DrawCount"() -> (w852:i32)
              n470 = Unbundle By Name(w838) -> ("status"=w859:bool)
              n471 = Equal To 0?(x=w836) -> (x = 0?=w837:bool)
              n472 = Concatenate Strings("WAIT FOR TOP HEATER AND COMP OFF.  " ("String"), w854, " checks." ("string")) -> (w856:string)
              n473 = local read "End Time(s)"() -> (w849:dbl)
              n474 = case shown="\"eHeat\"" w827 {
                tunnel: [w860 w861 w862] -> w828
                tunnel: w825 -> [w860 w861 _]
                tunnel: w824 -> [_ _ w862]
                frame "Hybrid", Default {
                }
                frame "StdElectric" {
                }
                frame "eHeat" {
                }
              }
              n475 = call "String_in_Reference.vi"("String"=w856) -> ()  [unwired: 18 in, 1 out]
              n476 = local read "t*=0"() -> (w851:dbl)
              n477 = local read "Stop Test"() -> (w833:bool)
              n478 = call "E-Time.vi"("error in (no error)"=w838) -> ("error out"=w858:errorcluster, "Elapsed Time (sec)"=w848:dbl)  [unwired: 8 in, 1 out]
              n479 = Subtract(x=w848, y=w851) -> (x-y=w850:dbl)
              n480 = Greater Than 0?(x=w852) -> (x > 0?=w847:bool)
              n481 = Greater?(x=w850, y=w849) -> (0:w846:bool)
              n482 = And(x=w847, y=w846) -> (x .and. y?=w845:bool)
              n483 = Compound Arithmetic op=AND(invert w833, invert w845, invert w859, w828, invert "Begin Draw") -> (w835:bool)
              n484 = Compound Arithmetic op=OR(w837, invert w835) -> (w834:bool)
              n485 = case shown="True" w834 {
                tunnel: w843 -> [_ w867]
                frame False {
                }
                frame True {
                  # "Record first and Last"
                  n486 = Index Array(array=w867, index (row)=1) -> (element=w868:string[])  [unwired: 1 in]
                  n487 = local read "FileName"() -> (w863:path)
                  n488 = call-poly <vilib>:"Write To Spreadsheet File.vi"("delimiter (\\t)"="," ("delimiter (\\t)"), "append to file? (new file:F)"=TRUE, "1D data"=w868, "file path (dialog if empty)"=w863) -> ()  [unwired: 4 in, 1 out]
                }
              }
            }
            n489 = case shown="False" w822 {
              tunnel: [w873 w875] -> w821
              tunnel: [w872 w878] -> w820
              tunnel: w819 -> [w872 w878]
              frame True {
                w873 = string[] ["Init Draw", "Draw", "Term Draw", "Finish"]  # States
                w871 = TRUE ("Special Last Draw")
                n490 = local write "Special Last Draw"(w871) -> ()
                n491 = local read "DrawCount"() -> (w870:i32)
                n492 = Increment(x=w870) -> (x+1=w869:i32)
                n493 = local write "DrawCount"(w869) -> ()
                "LastDraw" <- w871
              }
              frame False {
                w875 = string[] ["Init Draw", "Draw", "Term Draw", "Wait for Purge", "Purge", "Wait for Next Draw", "Finish"]  # States
                n494 = local read "DrawCount"() -> (w877:i32)
                n495 = Increment(x=w877) -> (x+1=w876:i32)
                n496 = local write "DrawCount"(w876) -> ()
                n497 = local write "Begin Draw"(FALSE ("Begin Draw")) -> ()
              }
            }
          }
        }
      }
      frame "Draw" {
        # "(For Last Draw, If after 30 sec, T< last tmin, stop and discard measurements, else continue)"
        n498 = while {
          shift-right: [w916] -> w882
          shift-left: w886 -> [w901]
          tunnel: w889 -> [w908]
          tunnel: [w908] -> w885
          shift-right: [w929] -> _
          shift-left: 15.0 ("GPM") -> [w928]
          shift-right: [w926] -> _
          shift-left: 0.0 ("GPM") -> [w925]
          tunnel: w884 -> [_]
          i -> [w918]
          stop <- w931 stop-if-true
          # "Sum of Temperatures"
          # "time to read"
          # "Start Special Case.  If after 30 sec, T< last\ntime, stop and discard measuremnts."
          # "Record output water temp after 15 secs, and at 5 sec intervals thereafter\nMonitor inlet water temp, must be 58 +/- 2 F\nTerminate draw when output temp = T*max -25F, record T*min"
          n499 = stacked-sequence {
            seq-local: [w933 _ _ _ _] -> [_ w944 w948 w951 w953]
            tunnel: w908 -> [w940 _ _ _ _]
            tunnel: [_ _ _ _ w952] -> w906
            tunnel: [_ w943 _ _ _] -> w903
            tunnel: [_ _ _ w951 _] -> w902
            tunnel: [w933 _ _ _ _] -> w900
            frame #0 {
              n500 = local read "Serial Data In"() -> (w937:string)
              n501 = local read "Label Array"() -> (w934:string[])
              n502 = local read "Chanel List"() -> (w938:string)
              n503 = local read "Equipment"() -> (w939:T6)
              n504 = control-ref of="Tank Display"() -> (w941:refnum<vi>)
              n505 = local read "Calibration File Array"() -> (w932:dbl[][])
              n506 = call "Gather Test Data - Heatup Test new.vi"("Agilent Scan List"=w938, "Semiphore"=w940, "Equipment"=w939, "Tank Display Ref"=w941, "Agilent?"=FALSE, "Calibration Coefficients"=w932, "Serial Data In"=w937, "Agilent Label Array"=w934) -> ("Output Data"=w933:string[][], "POWER"=w935:T3, "Voltage"=w936:dbl)  [unwired: 2 in, 3 out]
              n507 = local write "POWER"(w935) -> ()
              n508 = local write "Voltage"(w936) -> ()
              n509 = local write "Current Log Data"(w933) -> ()
            }
            frame #1 {
              n510 = call "Array_Search_For_Num.vi"("N Rows of Data"=w944, "Title?"="FLOW(GPM)" ("String")) -> ("number"=w943:dbl)  [unwired: 12 in, 1 out]
              "Flow" <- w943
              "FlowMeter During Draw" <- w943
              n511 = local read "Tank Display"() -> (w947:T4)
              n512 = Unbundle By Name(w947) -> ("TOUT"=→"RTD OUT":dbl)
            }
            frame #2 {
              n513 = call "Array_Search_For_Num.vi"("N Rows of Data"=w948, "Title?"="GALLONS") -> ("number"=→"M*(Gallons)":dbl)  [unwired: 12 in, 1 out]
            }
            frame #3 {
            }
            frame #4 {
              n514 = call "Array_Search_For_Num.vi"("N Rows of Data"=w953, "Title?"="Tc_down" ("String")) -> ("number"=w952:dbl)  [unwired: 12 in, 1 out]
            }
          }
          n515 = local read "Current Draw Start Time"() -> (w921:dbl)
          n516 = call "E-Time.vi"("error in (no error)"=w901) -> ("error out"=w927:errorcluster, "Elapsed Time (sec)"=w922:dbl)  [unwired: 8 in, 1 out]
          n517 = Subtract(x=w922, y=w921) -> (x-y=w899:dbl)
          "ETime" <- w899
          n518 = Greater Or Equal?(x=w899, y=w928) -> (x >= y?=w907:bool)
          n519 = case shown="True" w907 {
            tunnel: [w957 w997] -> w930
            tunnel: [w958 w996] -> w929
            tunnel: w928 -> [w958 w995]
            tunnel: w927 -> [w956 w974]
            tunnel: [w955 w994] -> w926
            tunnel: w925 -> [w955 w993]
            tunnel: [w957 w992] -> w924
            tunnel: [w957 w991] -> w923
            tunnel: w899 -> [_ _]
            tunnel: [w956 w980] -> w917
            tunnel: w908 -> [_ _]
            tunnel: w902 -> [_ w961]
            tunnel: w900 -> [_ w966]
            frame False {
              w957 = FALSE ("status")
            }
            frame True {
              # "assume last read is min."
              n520 = local read "Degree Setting"() -> (w981:dbl)
              n521 = local read "Temp Band(+/- F)"() -> (w982:dbl)
              n522 = local read "FileName"() -> (w969:path)
              n523 = Index Array(array=w966, index (row)=1) -> (element=w967:string[])  [unwired: 1 in]
              n524 = Add(x=5.0, y=w995) -> (x+y=w996:dbl)
              n525 = call "Array_Search_For_Num.vi"("N Rows of Data"=w961, "Title?"="RTD_IN" ("String")) -> ("number"=w975:dbl)  [unwired: 12 in, 1 out]
              "RTD_IN Value" <- w975
              n526 = call-poly <vilib>:"Write To Spreadsheet File.vi"("delimiter (\\t)"="," ("delimiter (\\t)"), "append to file? (new file:F)"=TRUE, "1D data"=w967, "file path (dialog if empty)"=w969) -> ()  [unwired: 4 in, 1 out]
              n527 = call "Array_Search_For_Num.vi"("N Rows of Data"=w961, "Title?"="RTD_OUT" ("String")) -> ("number"=w959:dbl)  [unwired: 12 in, 1 out]
              "T*min" <- w959
              n528 = local read "Special Last Draw"() -> (w983:bool)
              n529 = local read "Last T*min"() -> (w964:dbl)
              n530 = local read "Special Last Draw"() -> (w985:bool)
              n531 = Add(x=w981, y=w982) -> (x+y=w976:dbl)
              n532 = Subtract(x=w981, y=w982) -> (x-y=w977:dbl)
              n533 = In Range and Coerce(upper limit=w976, x=w975, lower limit=w977) -> (In Range?=w973:bool)  [unwired: 1 out]
              n534 = Equal?(x=35.0, y=w996) -> (x = y?=w986:bool)
              n535 = local read "T*max"() -> (w963:dbl)
              n536 = Max & Min(x=w963, y=w959) -> (max(x,y)=w965:dbl)  [unwired: 1 out]
              n537 = local write "T*max"(w965) -> ()
              n538 = Less?(x=w965, y=w964) -> (x < y?=w960:bool)
              n539 = Not(x=w973) -> (.not. x?=w972:bool)
              "Tin Fault" <- w972
              n540 = case shown="False" w983 {
                tunnel: [w999 w1001] -> w984
                frame False {
                  n541 = local read "T*max"() -> (w1000:dbl)
                  n542 = local read "TFall"() -> (w998:dbl)
                  n543 = Subtract(x=w1000, y=w998) -> (x-y=w999:dbl)
                }
                frame True {
                  n544 = local read "Last T*min"() -> (w1001:dbl)
                }
              }
              n545 = Compound Arithmetic op=AND(w960, w986, w985) -> (w991:bool)
              n546 = local write "Discard Last Draw"(w991) -> ()
              n547 = Add(x=w993, y=w959) -> (x+y=w994:dbl)
              n548 = call "Error Bool Enumerator.vi"("Error Enum"=HEWH_Error_Enumeration."RTD In Range Error", "Error In"=w974, "Error?"=w972) -> ("Error Out"=w980:errorcluster)  [unwired: 6 in]
              n549 = expression code="x/5-3"(w996) -> (w989:dbl)
              n550 = Unbundle By Name(w980) -> ("status"=w997:bool)
              n551 = Less Or Equal?(x=w959, y=w984) -> (x <= y?=w992:bool)
              n552 = Divide(x=w994, y=w989) -> (x/y=→"T*Ave":dbl)
            }
          }
          n553 = local read "Degree Setting"() -> (w910:dbl)
          n554 = local read "Temp Adj Draw"() -> (w904:dbl)
          n555 = local read "Flow Adj Draw"() -> (w905:dbl)
          n556 = local read "T5"() -> (w920:u32)
          n557 = local read "Flow rate setting"() -> (w914:dbl)
          n558 = local read "MW100"() -> (w915:refnum<visa-resource-name>)
          n559 = Wait (ms)(milliseconds to wait=w920) -> ()  [unwired: 1 out]
          n560 = Subtract(x=w910, y="RTD 2 Downspout offset") -> (x-y=w909:dbl)
          n561 = call "HEWH Flow and Temp Adjustment.vi"("MW100"=w915, "FlowReading"=w903, "Flow In"=w905, "K(0.1)"="K(0.1)", "TempReading"=w906, "Error In"=w917, "FlowTarget"=w914, "Temp Target"=w909, "Temp In"=w904, "Semiphore"=w908, "Elapsed Time (sec)"=w899, "Flow Adjust Time (3s)"="Flow Adjust Time (3s)") -> ("Flow Out"=→"Flow Adj Draw":dbl, "Temp Out"=→"Temp Adj Draw":dbl, "Error Out"=w916:errorcluster)  [unwired: 5 in]
          n562 = local read "Stop Test"() -> (w919:bool)
          n563 = Compound Arithmetic op=OR(w930, w924, w923, w919) -> (w931:bool)
          "Iteration" <- w918
        }
        n564 = case shown="No Error" w882 {
          selector: w882 -> [w890 w896]
          tunnel: [w892 string[] ["Finish"] ("States")] -> w883
          tunnel: w880 -> [w892 _]
          tunnel: [w891 w896] -> w881
          frame No Error {
            n565 = flat-sequence {
              tunnel: [w894] -> w891
              tunnel: w890 -> [w894]
              frame #0 {
                n566 = local write "Drawing"(FALSE) -> ()
              }
            }
          }
          frame Error {
          }
        }
      }
      frame "Term Draw" {
        # "Keep line pressure on tank."
        # "(For Last Draw, If after 30 sec, T< last tmin, stop and discard measurements, else continue)"
        # "Terminate draw.  Record Tmin*, Tmax*, Tave* and M*"
        n567 = local read "Expansion Tank?"() -> (w1008:bool)
        n568 = local read "MW100"() -> (w1017:refnum<visa-resource-name>)
        n569 = call "HEWH Set Valves.vi"("VISA session"=w1017, "Semiphore"=w1003, "Expansion Tank?"=w1008, "Valve Bank Setting"=ValveBankPositions."Heating", "Error In"=w1007) -> ("dup VISA session"=w1004:refnum<visa-resource-name>, "Error Out"=w1005:errorcluster)  [unwired: 9 in]
        n570 = local read "Discard Last Draw"() -> (w1011:bool)
        n571 = call "HEWH Totalize Flow Control.vi"("VISA session"=w1004, "Semiphore"=w1003, "Totalize Flow"=FALSE, "error in (no error)"=w1005) -> ("error out"=w1006:errorcluster)  [unwired: 10 in, 1 out]
        n572 = case shown="False" w1011 {
          tunnel: [w1034 w1040] -> w1013
          tunnel: w1012 -> [w1033 w1040]
          tunnel: [w1020 w1039] -> w1010
          tunnel: w1006 -> [w1032 w1039]
          tunnel: w1003 -> [w1029 _]
          frame False {
            n573 = local read "MW100"() -> (w1028:refnum<visa-resource-name>)
            n574 = local read "M*(Gallons)"() -> (w1035:dbl)
            n575 = local read "T*max"() -> (w1036:dbl)
            n576 = local read "T*Ave"() -> (w1037:dbl)
            n577 = local read "T*min"() -> (w1038:dbl)
            "Last T*min" <- w1038
            n578 = call "HEWH Read Power OhioSemitronics.vi"("VISA resource name"=w1028, "Semiphore"=w1029, "error in (no error)"=w1032) -> ("PowerData"=w1031:T24, "error out"=w1022:errorcluster)  [unwired: 9 in, 2 out]
            n579 = Unbundle By Name(w1031) -> ("WattHours"=w1030:dbl)
            "WattHours" <- w1030
            n580 = call "E-Time.vi"("error in (no error)"=w1022) -> ("error out"=w1020:errorcluster, "Elapsed Time (sec)"=w1021:dbl)  [unwired: 8 in, 1 out]
            n581 = Build Array(w1021, w1038, w1037, w1036, w1035, w1030) -> (w1027:dbl[])
            n582 = Number To Fractional String(number=w1027) -> (F-format string=w1025:string[])  [unwired: 3 in]
            n583 = Build Array (concatenate)(w1033, w1027) -> (w1034:dbl[][])
            n584 = Build Array (concatenate)("Draw Result(time;T*min;T*ave;T*max; M*gallons;WattHours)", w1025) -> (w1024:string[])
            n585 = local read "FileName"() -> (w1019:path)
            n586 = call-poly <vilib>:"Write To Spreadsheet File.vi"("delimiter (\\t)"="," ("delimiter (\\t)"), "append to file? (new file:F)"=TRUE, "1D data"=w1024, "file path (dialog if empty)"=w1019) -> ()  [unwired: 4 in, 1 out]
          }
          frame True {
          }
        }
        n587 = case shown="No Error" w1010 {
          selector: w1010 -> [w1041 w1044]
          tunnel: [w1042 string[] ["Finish"] ("States")] -> w1015
          tunnel: w1016 -> [w1042 _]
          tunnel: [w1041 w1044] -> w1014
          frame No Error {
          }
          frame Error {
          }
        }
      }
      frame "Finish", Default {
        n588 = local write "Tab Control"(8 ("index")) -> ()
        n589 = case shown="No Error" w1047 {
          selector: w1047 -> [w1061 w1064]
          tunnel: [w1062 w1067] -> w1058
          tunnel: w1057 -> [w1062 w1067]
          tunnel: [w1061 errorcluster {"status"=FALSE, "code"=0, "source"=""} ("error IO")] -> w1048
          frame No Error {
          }
          frame Error {
            n590 = Unbundle By Name(w1064) -> ("source"=w1063:string)
            n591 = local read "FileName"() -> (w1065:path)
            n592 = call "Log String to Spreadsheet.vi"("String"=w1063, "FileName"=w1065) -> ()  [unwired: 9 in, 1 out]
          }
        }
        n593 = Unbundle By Name(w1056) -> ("MW100"=w1049:refnum<visa-resource-name>)
        n594 = call "YKMW100 Get Error Log.vi"("VISA session"=w1049, "Semiphore"=w1046, "error in (no error)"=w1048) -> ("dup VISA session"=w1052:refnum<visa-resource-name>, "Error History"=→"Error History":string[], "error out"=w1053:errorcluster)  [unwired: 9 in, 1 out]
        n595 = call "YKMW100 Get Com Log.vi"("VISA session"=w1052, "Semiphore"=w1046, "error in (no error)"=w1053) -> ("Com History"=→"Com History":string[], "error out"=w1045:errorcluster)  [unwired: 9 in, 2 out]
        n596 = flat-sequence {
          tunnel: w1045 -> [_]
          frame #0 {
            w1060 = TRUE ("Stop Logging")
            n597 = local write "Stop Logging"(w1060) -> ()
            n598 = property on="Stop Logging" class="Bool (strict)"("Val(Sgnl)"=w1060) -> ()  [unwired: 2 in, 2 out]
            n599 = call "String_in_Reference.vi"("String"="Stopping Log") -> ()  [unwired: 18 in, 1 out]
          }
        }
      }
    }
    n600 = Build Array (concatenate)(w42, w37) -> (w41:string[])
    "Executaion Sequence" <- w41
    n601 = Equal?(x=w37, y="Finish") -> (x = y?=w51:bool)
    n602 = local read "T2"() -> (w43:u32)
    n603 = Wait (ms)(milliseconds to wait=w43) -> ()  [unwired: 1 out]
  }
  "Error Out" <- w9
  "Test Data" <- w11
  n604 = while {
    shift-right: [w1076] -> w7
    shift-left: w2 -> [w1077]
    shift-right: [w1068] -> _
    shift-left: 0.0 -> [w1069]
    stop <- w1070 stop-if-true
    # "Start Time of \nlast cycle"
    # "continuous data gathering"
    n605 = local read "Init Complete"() -> (w1074:bool)
    n606 = case shown="True" w1074 {
      tunnel: w1077 -> [w1079 w1096]
      tunnel: [w1079 w1097] -> w1076
      tunnel: [w1078 w1088] -> w1068
      tunnel: w1069 -> [w1078 w1083]
      frame False {
      }
      frame True {
        # "is time\nelapsed?"
        n607 = local read "End Time(s)"() -> (w1095:dbl)
        n608 = local read "Semiphore"() -> (w1080:T1)
        n609 = local read "t*=0"() -> (w1089:dbl)
        n610 = local read "t*=0"() -> (w1094:dbl)
        n611 = call "E-Time.vi"() -> ("Elapsed Time (sec)"=w1082:dbl)  [unwired: 9 in, 2 out]
        n612 = Increment(x=w1096) -> (x+1=w1097:i32)
        "Number of Records" <- w1097
        n613 = Multiply(x="Data Sample Period(10s)", y=1000.0) -> (x*y=w1085:dbl)
        n614 = Subtract(x=w1082, y=w1094) -> (x-y=w1093:dbl)
        n615 = To Long Integer(number=w1085) -> (32bit integer=w1084:i32)
        n616 = Greater Than 0?(x=w1089) -> (x > 0?=w1091:bool)
        n617 = Greater?(x=w1093, y=w1095) -> (0:w1090:bool)
        n618 = And(x=w1090, y=w1091) -> (x .and. y?=w1092:bool)
        n619 = call "RLT Timeout Calc.vi"("Complete time"=w1082, "Gather Data Period"=w1084, "Start Time"=w1083) -> ("coerced(x)"=w1081:i32)  [unwired: 8 in]
        n620 = case shown="True" w1092 {
          tunnel: w1080 -> [w1100 w1149]
          tunnel: [w1098 w1145] -> w1088
          tunnel: w1081 -> [w1099 w1144]
          frame False {
            n621 = event shown="[0] Timeout" {
              selector: _ -> [_]
              dyn-events: _ -> [_]
              timeout: w1099 -> [_]
              tunnel: w1100 -> [w1133]
              tunnel: [w1103] -> w1098
              event Timeout {
                n622 = event-data() -> ()  [unwired: 1 in, 2 out]
                n623 = flat-sequence {
                  tunnel: [w1143] -> w1105
                  tunnel: [w1142] -> w1103
                  frame #0 {
                    n624 = local read "Label Array"() -> (w1143:string[])
                    n625 = call "E-Time.vi"() -> ("Elapsed Time (sec)"=w1142:dbl)  [unwired: 9 in, 2 out]
                  }
                }
                n626 = local read "Serial Data In"() -> (w1106:string)
                n627 = local read "Chanel List"() -> (w1132:string)
                n628 = local read "Use Agilent?"() -> (w1107:bool)
                n629 = control-ref of="Tank Display"() -> (w1135:refnum<vi>)
                n630 = local read "Equipment"() -> (w1134:T6)
                n631 = local read "Drawing"() -> (w1102:bool)
                n632 = local read "Calibration File Array"() -> (w1101:dbl[][])
                n633 = call "Gather Test Data - Heatup Test new.vi"("Agilent Scan List"=w1132, "Semiphore"=w1133, "Equipment"=w1134, "Tank Display Ref"=w1135, "Agilent?"=w1107, "Calibration Coefficients"=w1101, "Serial Data In"=w1106, "Agilent Label Array"=w1105) -> ("Tc Tree"=w1118:dbl[], "Output Data"=w1109:string[][], "POWER"=w1120:T3, "PowerData"=w1121:T24, "Voltage"=w1104:dbl, "error out"=→"Error Datalogging":errorcluster)  [unwired: 2 in]
                "POWER" <- w1120
                n634 = Unbundle(w1120) -> ("UE"=w1123:bool, "LE"=w1125:bool, "COMP"=w1124:bool, "FANS"=w1119:bool)
                n635 = Boolean To (0,1)(Boolean=w1123) -> (0, 1=w1116:i16)
                n636 = Boolean To (0,1)(Boolean=w1119) -> (0, 1=w1110:i16)
                n637 = Boolean To (0,1)(Boolean=w1124) -> (0, 1=w1112:i16)
                n638 = Boolean To (0,1)(Boolean=w1125) -> (0, 1=w1114:i16)
                n639 = local write "Voltage"(w1104) -> ()
                n640 = Unbundle By Name(w1121) -> ("Power"=w1117:dbl)
                n641 = Array To Cluster(array=w1118) -> (cluster=w1130:T22)
                n642 = expression code="2*x"(w1112) -> (w1111:i16)
                n643 = expression code="3*x"(w1114) -> (w1113:i16)
                n644 = expression code="4*x"(w1116) -> (w1115:i16)
                n645 = call "Array_Search_For_Num.vi"("N Rows of Data"=w1109, "Title?"="GALLONS") -> ("number"=→"Gallons Chart":dbl)  [unwired: 12 in, 1 out]
                n646 = Build Array(w1130) -> (→"Temps":T8)
                n647 = Build Array(w1117, w1115, w1113, w1111, w1110) -> (w1128:dbl[])
                n648 = Array To Cluster(array=w1128) -> (cluster=w1126:T25)
                n649 = case shown="False" w1102 {
                  tunnel: w1109 -> [w1136 _]
                  frame False {
                    n650 = local read "FileName"() -> (w1141:path)
                    n651 = Index Array(array=w1136, index (row)=1) -> (element=w1139:string[])  [unwired: 1 in]
                    n652 = call-poly <vilib>:"Write To Spreadsheet File.vi"("delimiter (\\t)"="," ("delimiter (\\t)"), "append to file? (new file:F)"=TRUE, "1D data"=w1139, "file path (dialog if empty)"=w1141) -> ()  [unwired: 4 in, 1 out]
                    "Current Log Data" <- w1136
                  }
                  frame True {
                  }
                }
                n653 = Build Array(w1126) -> (→"Watt Chart":T10)
              }
            }
          }
          frame True {
            w1151 = T26 30 items=["4-20_OUT", "Pres_HI1", "Pres_HI2", "Pres_LOW", "Pres_PIN", "HEATER_TOP", "HEATER_BOT", "T_Shell", "FLOWMETER", "WATT_SENSE", "WH_TICK", "Tc_1", "Tc_2", "Tc_3", "Tc_4", "Tc_5", "Tc_6", "Tc_down", "T_Shell_2", "T_Shell_3", "T_Shell_4", "RTD_IN", "RTD_OUT", "RTD_AMB", "INTF_TEMPFLO", "INTF_READY", "INTF_START", "INTF_STOP", "DRM_LOW", "DRM_HIGH", "PWR_MAIN", "VLV_DUMP", "VLV_OUT", "VLV_IN", "WATT_HOURS", "FLOW(SAMPLE)", "GALLONS", "FLOW(GPM)"] ("Channel_Enum")
            # "Over Time Limit, Turn off Power"
            n654 = local read "MW100"() -> (w1148:refnum<visa-resource-name>)
            n655 = call "YKMW100 VF0 Relay Status.vi"("VISA session"=w1148, "Semiphore"=w1149, "Channel_Enum"=w1151) -> ("dup VISA session"=w1147:refnum<visa-resource-name>, "Output On"=w1150:bool, "error out"=w1146:errorcluster)  [unwired: 9 in, 1 out]
            n656 = case shown="False" w1150 {
              tunnel: w1149 -> [w1155 w1201]
              tunnel: w1147 -> [_ w1202]
              tunnel: w1146 -> [w1154 w1189]
              tunnel: [w1152 w1180] -> w1145
              tunnel: w1144 -> [w1153 _]
              frame True {
                n657 = event shown="[0] Timeout" {
                  selector: _ -> [_]
                  dyn-events: _ -> [_]
                  timeout: w1153 -> [_]
                  tunnel: w1155 -> [w1170]
                  tunnel: w1154 -> [w1168]
                  tunnel: [w1158] -> w1152
                  event Timeout {
                    # "Only reccord the required\ndata during the draw."
                    # "Power is off."
                    n658 = event-data() -> ()  [unwired: 1 in, 2 out]
                    n659 = local read "Serial Data In"() -> (w1161:string)
                    n660 = flat-sequence {
                      tunnel: [w1178] -> w1159
                      tunnel: [w1177] -> w1158
                      frame #0 {
                        n661 = local read "Label Array"() -> (w1178:string[])
                        n662 = call "E-Time.vi"() -> ("Elapsed Time (sec)"=w1177:dbl)  [unwired: 9 in, 2 out]
                      }
                    }
                    n663 = local read "Use Agilent?"() -> (w1162:bool)
                    n664 = control-ref of="Tank Display"() -> (w1172:refnum<vi>)
                    n665 = local read "Chanel List"() -> (w1164:string)
                    n666 = local read "Equipment"() -> (w1171:T6)
                    n667 = local read "Calibration File Array"() -> (w1156:dbl[][])
                    n668 = call "Gather Test Data - Heatup Test new.vi"("Agilent Scan List"=w1164, "Semiphore"=w1170, "Equipment"=w1171, "Tank Display Ref"=w1172, "Agilent?"=w1162, "Calibration Coefficients"=w1156, "error in (no error)"=w1168, "Serial Data In"=w1161, "Agilent Label Array"=w1159) -> ("Output Data"=w1166:string[][], "POWER"=w1169:T3, "Voltage"=w1160:dbl, "error out"=w1163:errorcluster)  [unwired: 1 in, 2 out]
                    n669 = local write "Voltage"(w1160) -> ()
                    n670 = local write "Current Log Data"(w1166) -> ()
                    n671 = local write "POWER"(w1169) -> ()
                    n672 = local write "Error Datalogging"(w1163) -> ()
                    n673 = local read "Drawing"() -> (w1157:bool)
                    n674 = Index Array(array=w1166, index (row)=1) -> (element=w1165:string[])  [unwired: 1 in]
                    n675 = case shown="False" w1157 {
                      tunnel: w1165 -> [w1176 _]
                      frame False {
                        n676 = local read "FileName"() -> (w1175:path)
                        n677 = call-poly <vilib>:"Write To Spreadsheet File.vi"("delimiter (\\t)"="," ("delimiter (\\t)"), "append to file? (new file:F)"=TRUE, "1D data"=w1176, "file path (dialog if empty)"=w1175) -> ()  [unwired: 4 in, 1 out]
                      }
                      frame True {
                      }
                    }
                  }
                }
              }
              frame False {
                w1200 = T26 30 items=["4-20_OUT", "Pres_HI1", "Pres_HI2", "Pres_LOW", "Pres_PIN", "HEATER_TOP", "HEATER_BOT", "T_Shell", "FLOWMETER", "WATT_SENSE", "WH_TICK", "Tc_1", "Tc_2", "Tc_3", "Tc_4", "Tc_5", "Tc_6", "Tc_down", "T_Shell_2", "T_Shell_3", "T_Shell_4", "RTD_IN", "RTD_OUT", "RTD_AMB", "INTF_TEMPFLO", "INTF_READY", "INTF_START", "INTF_STOP", "DRM_LOW", "DRM_HIGH", "PWR_MAIN", "VLV_DUMP", "VLV_OUT", "VLV_IN", "WATT_HOURS", "FLOW(SAMPLE)", "GALLONS", "FLOW(GPM)"] ("Channel_Enum")
                # "Turn Off Power"
                n678 = local read "FileName"() -> (w1187:path)
                n679 = flat-sequence {
                  tunnel: [w1206] -> w1181
                  tunnel: [w1205] -> w1180
                  frame #0 {
                    n680 = local read "Label Array"() -> (w1206:string[])
                    n681 = call "E-Time.vi"() -> ("Elapsed Time (sec)"=w1205:dbl)  [unwired: 9 in, 2 out]
                  }
                }
                n682 = call "Log String to Spreadsheet.vi"("String"="Turn off Power ", "error in (no error)"=w1189, "FileName"=w1187) -> ("error out"=w1188:errorcluster)  [unwired: 8 in]
                n683 = local read "Serial Data In"() -> (w1183:string)
                n684 = local read "Use Agilent?"() -> (w1184:bool)
                n685 = call "Generic - DO1.vi"("VISA session"=w1202, "Semiphore"=w1201, "Channel_Enum"=w1200, "Relay Status (0:CLOSED)"=enum8{"CLOSED", "OPEN"}."CLOSED", "Error In"=w1188) -> ("error out"=w1195:errorcluster)  [unwired: 9 in, 1 out]
                n686 = local read "Chanel List"() -> (w1191:string)
                n687 = control-ref of="Tank Display"() -> (w1204:refnum<vi>)
                n688 = local read "Equipment"() -> (w1203:T6)
                n689 = local read "Calibration File Array"() -> (w1179:dbl[][])
                n690 = call "Gather Test Data - Heatup Test new.vi"("Agilent Scan List"=w1191, "Semiphore"=w1201, "Equipment"=w1203, "Tank Display Ref"=w1204, "Agilent?"=w1184, "Calibration Coefficients"=w1179, "error in (no error)"=w1195, "Serial Data In"=w1183, "Agilent Label Array"=w1181) -> ("Output Data"=w1193:string[][], "POWER"=w1190:T3, "Voltage"=w1182:dbl, "error out"=w1185:errorcluster)  [unwired: 1 in, 2 out]
                n691 = local write "POWER"(w1190) -> ()
                n692 = local write "Current Log Data"(w1193) -> ()
                n693 = local write "Error Datalogging"(w1185) -> ()
                n694 = local write "Voltage"(w1182) -> ()
                n695 = Index Array(array=w1193, index (row)=1) -> (element=w1192:string[])  [unwired: 1 in]
                n696 = local read "FileName"() -> (w1198:path)
                n697 = call-poly <vilib>:"Write To Spreadsheet File.vi"("delimiter (\\t)"="," ("delimiter (\\t)"), "append to file? (new file:F)"=TRUE, "1D data"=w1192, "file path (dialog if empty)"=w1198) -> ()  [unwired: 4 in, 1 out]
              }
            }
          }
        }
      }
    }
    n698 = local read "T2"() -> (w1075:u32)
    n699 = Wait (ms)(milliseconds to wait=w1075) -> ()  [unwired: 1 out]
    n700 = local read "Error Datalogging"() -> (w1073:errorcluster)
    n701 = Unbundle By Name(w1073) -> ("status"=w1071:bool)
    n702 = Or(x="Stop Logging", y=w1071) -> (x .or. y?=w1070:bool)
  }
  n703 = disable-structure shown="Enabled" {
    frame Enabled {
      n704 = event shown="[1] \"Init Complete\", \"Stop Logging\": Value Change" {
        selector: _ -> [_ _]
        dyn-events: _ -> [_ _]
        timeout: _ -> [_ _]
        event Timeout {
          n705 = event-data() -> ()  [unwired: 1 in, 2 out]
        }
        event "Init Complete", "Stop Logging": Value Change {
          # "Gather Serial Data Routine."
          n706 = event-data() -> ()  [unwired: 1 in, 5 out]
          n707 = local read "COM Port"() -> (w1209:refnum<visa-resource-name>)
          n708 = local read "Serial Port Available?"() -> (w1207:bool)
          n709 = while {
            tunnel: w1209 -> [w1216]
            tunnel: ["StopSerial"] -> w1208
            tunnel: w1207 -> [w1212]
            stop <- "StopSerial" stop-if-true
            n710 = local read "GEA2 HyperData"() -> (w1213:bool)
            n711 = case shown="True" w1212 {
              tunnel: w1216 -> [_ w1223]
              tunnel: w1213 -> [_ w1218]
              frame False {
              }
              frame True {
                n712 = Select(t=10, s=w1218, f=1) -> (s? t:f=w1219:i32)
                n713 = call "HEWH Serial Data Read.vi"("Serial Port Ref"=w1223, "GEA2 HyperData"=w1218, "Retries"=w1219) -> ("Serial Read OK"=w1217:bool, "Read String"=w1224:string, "error out"=→"Error Serial":errorcluster)  [unwired: 9 in, 1 out]
                n714 = case shown="False" w1217 {
                  frame False {
                    n715 = call "Counter.vi"() -> ("Count"=→"Com Errs":dbl)  [unwired: 11 in]
                  }
                  frame True {
                  }
                }
                n716 = local write "Serial Data In"(w1224) -> ()
              }
            }
            n717 = Wait (ms)(milliseconds to wait=u32 500) -> ()  [unwired: 1 out]
          }
          n718 = flat-sequence {
            tunnel: w1208 -> [_]
            frame #0 {
              w1211 = TRUE ("stop")
              n719 = property on="Stop" class="Bool (strict)"("Val(Sgnl)"=w1211) -> ()  [unwired: 2 in, 2 out]
              n720 = local write "Stop"(w1211) -> ()
              n721 = call "String_in_Reference.vi"("String"="Stopping Test") -> ()  [unwired: 18 in, 1 out]
            }
          }
        }
      }
    }
    frame Disabled {
    }
  }
  n722 = flat-sequence {
    tunnel: w7 -> [_]
    frame #0 {
      w1227 = TRUE ("stop")
      n723 = local write "StopSerial"(w1227) -> ()
      n724 = property on="StopSerial" class="Bool (strict)"("Val(Sgnl)"=w1227) -> ()  [unwired: 2 in, 2 out]
      n725 = call "String_in_Reference.vi"("String"="Stopping Serial Port") -> ()  [unwired: 18 in, 1 out]
    }
  }
  n726 = disable-structure shown="Enabled" {
    frame Enabled {
      n727 = while {
        stop <- w1229 stop-if-true
        n728 = local read "T3"() -> (w1228:u32)
        n729 = event shown="[1] \"Stop\": Value Change" {
          selector: _ -> [_ _ _ _]
          dyn-events: _ -> [_ _ _ _]
          timeout: w1228 -> [_ _ _ _]
          tunnel: [_ w1232 _ _] -> w1229
          event Timeout {
            n730 = event-data() -> ()  [unwired: 1 in, 2 out]
            n731 = call "String_in_Reference.vi"() -> ("String Out"=→"STATUS":string)  [unwired: 19 in]
            n732 = call "E-Time.vi"() -> ("Elapsed Time (sec)"=→"Elapsed Time (sec)":dbl)  [unwired: 9 in, 2 out]
          }
          event "Stop": Value Change {
            n733 = event-data() -> ()  [unwired: 1 in, 5 out]
            n734 = case shown="True" "Stop" {
              tunnel: [_ w1234] -> w1232
              frame False {
              }
              frame True {
                n735 = stacked-sequence {
                  tunnel: [_ _ _ _ _ _ _ _ TRUE ("stop? (T)")] -> w1234
                  frame #0 {
                    w1239 = T26 30 items=["4-20_OUT", "Pres_HI1", "Pres_HI2", "Pres_LOW", "Pres_PIN", "HEATER_TOP", "HEATER_BOT", "T_Shell", "FLOWMETER", "WATT_SENSE", "WH_TICK", "Tc_1", "Tc_2", "Tc_3", "Tc_4", "Tc_5", "Tc_6", "Tc_down", "T_Shell_2", "T_Shell_3", "T_Shell_4", "RTD_IN", "RTD_OUT", "RTD_AMB", "INTF_TEMPFLO", "INTF_READY", "INTF_START", "INTF_STOP", "DRM_LOW", "DRM_HIGH", "PWR_MAIN", "VLV_DUMP", "VLV_OUT", "VLV_IN", "WATT_HOURS", "FLOW(SAMPLE)", "GALLONS", "FLOW(GPM)"] ("Channel_Enum")
                    # "Turn off water, and power on, open output valve."
                    n736 = local read "Semiphore"() -> (w1238:T1)
                    n737 = local read "Expansion Tank?"() -> (w1237:bool)
                    n738 = local read "MW100"() -> (w1235:refnum<visa-resource-name>)
                    n739 = call "HEWH Set Valves.vi"("VISA session"=w1235, "Semiphore"=w1238, "Expansion Tank?"=w1237, "Valve Bank Setting"=ValveBankPositions."Resting") -> ("dup VISA session"=w1242:refnum<visa-resource-name>, "Error Out"=w1241:errorcluster)  [unwired: 10 in]
                    n740 = call "Generic - DO1.vi"("VISA session"=w1242, "Semiphore"=w1238, "Channel_Enum"=w1239, "Relay Status (0:CLOSED)"=enum8{"CLOSED", "OPEN"}."OPEN", "Error In"=w1241) -> ()  [unwired: 9 in, 2 out]
                  }
                  frame #1 {
                    n741 = local read "Stop Test"() -> (w1243:bool)
                    n742 = case shown="True" w1243 {
                      frame False {
                      }
                      frame True {
                        n743 = local read "FileName"() -> (w1244:path)
                        n744 = call "Log String to Spreadsheet.vi"("String"="Stop Button Pressed", "FileName"=w1244) -> ()  [unwired: 9 in, 1 out]
                      }
                    }
                  }
                  frame #2 {
                    n745 = local read "Com Errs"() -> (w1250:dbl)
                    n746 = To Unsigned Long Integer(number=w1250) -> (unsigned 32bit integer=w1248:u32)
                    n747 = Number To Decimal String(number=w1248) -> (decimal integer string=w1246:string)  [unwired: 1 in]
                    n748 = Concatenate Strings("Com Errors: " ("String"), w1246) -> (w1249:string)
                    n749 = local read "FileName"() -> (w1251:path)
                    n750 = call "Log String to Spreadsheet.vi"("String"=w1249, "FileName"=w1251) -> ()  [unwired: 9 in, 1 out]
                  }
                  frame #3 {
                    n751 = local read "Error Datalogging"() -> (w1253:errorcluster)
                    n752 = Unbundle By Name(w1253) -> ("status"=w1252:bool)
                    n753 = case shown="True" w1252 {
                      frame False {
                      }
                      frame True {
                        n754 = local read "FileName"() -> (w1254:path)
                        n755 = call "Log String to Spreadsheet.vi"("String"="Error Data Logging", "FileName"=w1254) -> ()  [unwired: 9 in, 1 out]
                      }
                    }
                  }
                  frame #4 {
                    n756 = local read "Init Complete"() -> (w1257:bool)
                    n757 = local read "Local?"() -> (w1256:bool)
                    n758 = And(x=w1256, y=w1257) -> (x .and. y?=w1258:bool)
                    n759 = case shown="True" w1258 {
                      tunnel: w1256 -> [_ w1259]
                      frame False {
                      }
                      frame True {
                        n760 = local read "Equipment"() -> (w1262:T6)
                        n761 = local read "Semiphore"() -> (w1261:T1)
                        n762 = call "HEWH CloseEquipmet.vi"("Semiphore"=w1261, "Equipment"=w1262) -> ("Error Out"=w1260:errorcluster)  [unwired: 9 in]
                        n763 = call "Semiphore-Destroy-Local.vi"("Semiphore"=w1261, "Local?"=w1259, "error in (no error)"=w1260) -> ()  [unwired: 16 in, 1 out]
                      }
                    }
                  }
                  frame #5 {
                    n764 = local read "FileName"() -> (w1264:path)
                    n765 = call <vilib>:"Check if File or Folder Exists.vi"("path"=w1264) -> ("file or folder exists?"=w1263:bool)  [unwired: 8 in, 2 out]
                    n766 = case shown="True" w1263 {
                      tunnel: w1264 -> [_ w1272]
                      frame False {
                      }
                      frame True {
                        n767 = Strip Path(path=w1272) -> (name=w1271:string)  [unwired: 1 out]
                        n768 = Search and Replace String(input string=w1271, search string=".tmp", replace string=".csv" ("search string")) -> (result string=w1269:string, error out=w1275:errorcluster)  [unwired: 5 in, 2 out]
                        n769 = Build Path(base path="Save File Directory", name or relative path=w1269) -> (appended path=w1268:path)
                        n770 = Move(source path=w1272, error in=w1275, 10:w1268) -> (error out=w1267:errorcluster, 3:w1266:path)  [unwired: 2 in, 1 out]
                        n771 = local write "FileName"(w1268) -> ()
                        n772 = Set Permissions(7:i16 0 ("permissions"), 8:w1267, 11:w1266) -> ()  [unwired: 2 in, 2 out]
                      }
                    }
                  }
                  frame #6 {
                    n773 = event shown="[1] \"StopSerial\": Value Change" {
                      selector: _ -> [_ _]
                      dyn-events: _ -> [_ _]
                      timeout: _ -> [_ _]
                      event Timeout {
                        n774 = event-data() -> ()  [unwired: 1 in, 2 out]
                      }
                      event "StopSerial": Value Change {
                        w1276 = FALSE ("stop")
                        n775 = event-data() -> ()  [unwired: 1 in, 2 out]
                        n776 = local write "Stop"(w1276) -> ()
                        n777 = local write "Stop Logging"(w1276) -> ()
                        n778 = local write "STATUS"("Stopped OK." ("STATUS")) -> ()
                        n779 = local write "Stop Test"(w1276) -> ()
                      }
                    }
                  }
                  frame #7 {
                    w1278 = ","
                    n780 = local read "Computer Name"() -> (w1284:string)
                    n781 = local read "Ver."() -> (w1283:string)
                    n782 = property class="App"() -> ("App.Name"=w1281:string)  [unwired: 2 in, 2 out]
                    n783 = local read "LAN IP Address"() -> (w1280:string)
                    n784 = Concatenate Strings(w1280, w1278, w1284, w1278, w1281, w1278, w1283, w1278, "Completed." ("string")) -> (w1279:string)
                    n785 = call "Save Time to File.vi"("String"=w1279) -> ()  [unwired: 13 in, 2 out]
                  }
                  frame #8 {
                    n786 = local read "exe?"() -> (w1285:bool)
                    n787 = case shown="True" w1285 {
                      frame False {
                      }
                      frame True {
                        n788 = global read "Global HEWH.vi" "Test Station:"() -> (w1289:string)
                        n789 = Concatenate Strings("robocopy c:/Data //10.2.0.10/AP2Lab/" ("command line"), w1289) -> (w1290:string)
                        n790 = call <vilib>:"System Exec.vi"("run minimized? (F)"=TRUE, "command line"=w1290) -> ()  [unwired: 6 in, 4 out]
                      }
                    }
                  }
                }
              }
            }
          }
          event "Error Datalogging.status": Value Change {
            n791 = event-data() -> ()  [unwired: 1 in, 5 out]
            n792 = local read "Error Datalogging"() -> (w1292:errorcluster)
            n793 = Unbundle By Name(w1292) -> ("status"=w1291:bool)
            n794 = case shown="True" w1291 {
              frame False {
              }
              frame True {
                n795 = local read "FileName"() -> (w1293:path)
                n796 = call "Log String to Spreadsheet.vi"("String"="Error Logging Data", "FileName"=w1293) -> ()  [unwired: 9 in, 1 out]
              }
            }
          }
          event "Help": Value Change {
            n797 = event-data() -> ()  [unwired: 1 in, 5 out]
            n798 = One Button Dialog(message="\n10 CFR part 430 5.1.4 First-Hour Rating Test\n5.1.4.3.P1.2\tWater heater not operating, initiate a draw\n5.1.4.3.P1.3\tTerminate draw after cut in of the upper most element\n5.1.4.3.P1.4\tAfter cut out, monitor 6 internal Tcs every minute\n5.1.4.3.P2.1\tInitiate draw After cut out and average tank temp is max\n5.1.4.3.P2.2\tRecord output water temp after 15 secs, and at 5 sec intervals thereafter\n5.1.4.3.P2.3\tMonitor inlet water temp, must be 58 +/- 2 F\n5.1.4.3.P2.4\tTerminate draw when ouytput temp = T*max -25F, record T*min\n5.1.4.3.P2.5\tRecord ave output water temp, Mass/volumt removed\n5.1.4.3.P3.1\tPerform second draw when eletricity to heating is reduced\n5.1.4.3.P4\tRepeat for 1 hour\n\tLast draw: there are special cases\n5.1.4.3.P5.1\tA  draw is going at t-1 hr, complete\n5.1.4.3.P5.1.5\tIf a draw is not going, immediately start and continue for at least 30 seconds\n5.1.4.3.P5.1.6\t If after 30 sec, T< last tmin, stop and discard measurements, else continue\n") -> (true=w1296:bool)  [unwired: 1 in]
            n799 = Not(x=w1296) -> (.not. x?=w1295:bool)
            n800 = local write "Help"(w1295) -> ()
          }
        }
      }
    }
    frame Disabled {
    }
  }
